vi "电机控制上位机 - 副本.vi"() -> ()   [LabVIEW 2018]
uses:
  <vilib>/Instr/_visa.llb/VISA Set IO Buffer Mask.ctl
  <vilib>/Instr/_visa.llb/VISA Configure Serial Port (Instr).vi
panel:
  in  "VISA resource name":refnum<visa-resource-name> caption="串口号"
  in  "目标速度Motor2":i16(slide) scale=-1000.0..1000.0
  in  "目标速度Motor1":i16(slide) step=100 scale=-1000.0..1000.0 scale format="%10d"
  out "数值 5":i32
  out "数值 4":u8
  out "无符号字节数组":u8[](array[numeric])
  out "数值 3":dbl
  out "布尔":bool
  out "目标速度2":i32
  out "值":enum32{"力矩模式", "速度模式", "位置模式"}(ring)
  in  "数值 2":i8
  in  "位置取反":bool
  out "目标速度 1":i32
  in  "弧度脉冲":bool
  out "数值":u8
  in  "运动控制":bool
  in  "串口设置":bool
  in  "示波器":bool
  in  "电机2":bool
  in  "电机1":bool
  in  "参数监控":bool
  in  "选项卡控件":T1(tab)
  in  "保存数据":bool
  in  "清空显示":bool
  out "字符串":string
  in  "参数下发":bool
  out "数      据      显      示":string
  in  "Flash保存":bool
  in  "串口号":refnum<visa-resource-name>="COM4"
  in  "波特率":u32(ring)=115200 items=["9600"=9600, "19200"=19200, "115200"=115200, "128000"=128000, "256000"=256000, "460800"=460800]
  in  "数据位":u16(ring)=8 items=["5"=5, "6"=6, "7"=7, "8"=8]
  in  "校验位":u16(ring) items=["None", "Odd", "Even", "Mark", "Space", ""]
  in  "停止位":u16(ring)=10 items=["1.0"=10, "1.5"=15, "2.0"=20]
  in  "打开/关闭串口":bool
  in  "参数上传":bool
  out "电机2状态":u32(ring) items=["无错误"=0, "FOC执行错误"=1, "过压"=2, "欠压"=4, "过温"=8, "霍尔错误"=16, "速度反馈错误"=32, "短路保护"=64, "软件错误"=128, "1_3倍过载"=256, "1_5倍过载"=512, "电机过流"=1024, "刹车电阻开启"=2048, "电机堵转"=4096, "电机失速"=8192, "位置跟随错误"=16384, "霍尔学习错误"=32768, "CAN通信错误"=65536, "电机缺相"=131072]
  out "电机2温度":i32(slide) scale=0.0..150.0
  out "电机1温度":i32(slide) scale=0.0..150.0
  out "母线电压":i32(knob) scale=0.0..50.0
  out "电机2实际位置":i32(knob) scale=-2147483647.0..2147483647.0
  out "电机2实际电流":i32(knob) scale=-20000.0..20000.0
  out "电机2实际速度":i32(knob) scale=-5000.0..5000.0
  out "电机1实际位置":i32(knob) scale=-2147483647.0..2147483647.0
  out "电机1实际电流":i32(knob) scale=-20000.0..20000.0
  out "电机1实际速度":i32(knob) scale=-5000.0..5000.0
  out "电机1状态":u32(ring) items=["无错误"=0, "FOC执行错误"=1, "过压"=2, "欠压"=4, "过温"=8, "霍尔错误"=16, "速度反馈错误"=32, "短路保护"=64, "软件错误 "=128, "1_3倍过载"=256, "1_5倍过载"=512, "电机过流"=1024, "刹车电阻开启"=2048, "电机堵转"=4096, "电机失速"=8192, "位置跟随错误"=16384, "霍尔学习错误"=32768, "CAN通信错误"=65536, "电机缺相"=131072]
  in  "写入3":bool
  in  "读取 3":bool
  in  "ID 3":u8
  in  "数值3":i32 caption="数值"
  in  "DIV1":u32
  in  "锁相环1":bool
  in  "Ppll":u32
  in  "Ipll":u32
  in  "发送保护参数":bool
  in  "堵转时间":i32
  in  "堵转电流":i32
  in  "堵转速度":i32
  in  "最大速度":i32
  in  "最大相电流":i32
  in  "峰值电流持续时间":i32
  in  "电机峰值电流":i32
  in  "发送电机参数":bool
  in  "编码器分辨率":u32
  in  "额定转速":i32
  in  "额定转矩":i32
  in  "额定电流":i32
  in  "电机惯量":i32
  in  "力矩常数":i32
  in  "Pairs":i32
  in  "Pc1":u32
  in  "Ic 1":u32
  in  "Pv1":u32
  in  "Iv 1":u32
  in  "Pp 1":u32
  in  "Ip 1":u32
  in  "发送 PID 1":bool
  in  "Dp1":u32
  in  "写入2":bool
  in  "读取 2":bool
  in  "ID 2":u8
  in  "数值2":i32 caption="数值"
  in  "DIV2":u32
  in  "锁相环2":bool
  in  "Ppll 2":u32 caption="Ppll"
  in  "Ipll 2":u32
  in  "Dp2":u32
  in  "发送 PID 2":bool
  in  "Ip 2":u32
  in  "Pp2":u32
  in  "Iv 2":u32
  in  "Pv 2":u32
  in  "Ic2":u32
  in  "Pc 2":u32
  in  "Pairs 2":i32
  in  "力矩常数 2":i32
  in  "电机惯量 2":i32
  in  "额定电流 2":i32
  in  "额定转矩 2":i32
  in  "额定转速 2":i32
  in  "编码器分辨率 2":i32
  in  "发送电机参数 2":bool
  in  "电机峰值电流 2":i32
  in  "峰值电流持续时间 2":i32
  in  "最大相电流 2":i32
  in  "最大速度 2":i32
  in  "堵转速度 2":i32
  in  "堵转电流 2":i32
  in  "堵转时间 2":i32
  in  "发送保护参数 2":bool
  in  "同步模式开关":bool
  in  "写入":bool
  in  "读取":bool
  in  "ID":u8
  in  "数值1":i32 caption="数值"
  in  "确认换向参数":bool
  in  "换向电流":i32
  in  "确认电机":bool
  in  "确定运行模式":bool
  in  "执行换向":bool
  in  "电机失能":bool
  in  "运行模式":enum32{"力矩模式", "速度模式", "位置模式"}(tab)
  in  "目标力矩Motor 2":i32
  in  "下发力矩参数":bool
  in  "目标力矩Motor 1":i32
  in  "目标时间Motor2":i32
  in  "目标速度Motor2":i32
  in  "目标时间Motor1":i32
  in  "目标速度Motor1":i32
  in  "下发速度参数":bool
  in  "目标位置Motor2":i32
  in  "目标加速度Motor2":i32
  in  "目标减速度Motor2":i32
  in  "目标速度Motor2":i32
  in  "下发位置参数":bool
  in  "目标位置Motor1":i32
  in  "目标加速度Motor1":i32
  in  "目标减速度Motor1":i32
  in  "目标速度Motor1":i32
  in  "换向模式":string(combo)="1"
  in  "Motor1":bool
  in  "Motor2":bool
  in  "电机使能":bool
  in  "急停":bool
  in  "运行模式1":string(combo)="2"
  out "数值1 2":i32 caption="数值" format="%x"
  in  "报警清除":bool
  in  "参数确定":bool
  in  "确认ID":bool
  in  "参数4":u8(ring) items=["电机1参考电流", "电机1实际电流", "电机1参考速度", "电机1实际速度", "电机1参考位置", "电机1实际位置", "电机2参考电流", "电机2实际电流", "电机2参考速度", "电机2实际速度", "电机2参考位置", "电机2实际位置", ""]
  in  "参数3":u8(ring) items=["电机1参考电流", "电机1实际电流", "电机1参考速度", "电机1实际速度", "电机1参考位置", "电机1实际位置", "电机2参考电流", "电机2实际电流", "电机2参考速度", "电机2实际速度", "电机2参考位置", "电机2实际位置", ""]
  in  "参数2":T2(ring)
  in  "参数1":u8(ring) items=["电机1参考电流", "电机1实际电流", "电机1参考速度", "电机1实际速度", "电机1参考位置", "电机1实际位置", "电机2参考电流", "电机2实际电流", "电机2参考速度", "电机2实际速度", "电机2参考位置", "电机2实际位置", ""]
  in  "ID 4":u8
  in  "ID 3":u8
  in  "ID 2":u8
  in  "ID 1":u8
  out "波形图表":cluster{i32, i32, i32, i32}(graph)
  in  "停止":bool
  # "电机极对数"
  # "pairs"
  # "峰值电流"
  # "mA"
  # "mNm/A"
  # "ms"
  # "力矩常数"
  # "峰值时间"
  # "电机惯量"
  # "Kgm2"
  # "最大相电流"
  # "mA"
  # "rpm"
  # "额定电流"
  # "mA"
  # "最大速度"
  # "mNm"
  # "rpm"
  # "额定转矩"
  # "堵转速度"
  # "额定转速"
  # "rpm"
  # "堵转电流"
  # "mA"
  # "编码器分辨率"
  # "counts/r"
  # "堵转时间"
  # "ms"
  # "电流环"
  # "Pc"
  # "位置环"
  # "Ppll"
  # "Pp"
  # "Ic"
  # "Ip"
  # "Ipll"
  # "速度环"
  # "DIV"
  # "Dp"
  # "Pv"
  # "Iv"
  # "独立参数读取"
  # "pairs"
  # "mA"
  # "电机极对数"
  # "峰值电流"
  # "mNm/A"
  # "力矩常数"
  # "ms"
  # "峰值时间"
  # "Kgm2"
  # "电机惯量"
  # "mA"
  # "最大相电流"
  # "mA"
  # "rpm"
  # "额定电流"
  # "最大速度"
  # "mNm"
  # "额定转矩"
  # "rpm"
  # "堵转速度"
  # "rpm"
  # "额定转速"
  # "mA"
  # "堵转电流"
  # "counts/r"
  # "编码器分辨率"
  # "ms"
  # "堵转时间"
  # "电流环"
  # "位置环"
  # "Pc"
  # "Pp"
  # "Ppll"
  # "Ic"
  # "Ip"
  # "速度环"
  # "Ipll"
  # "Pv"
  # "Dp"
  # "DIV"
  # "Iv"
  # "独立参数读取"
  # "电机选择"
  # "独立参数读取"
  # "mA"
  # "mNm"
  # "mNm"
  # "rpm"
  # "ms"
  # "rpm"
  # "ms"
  # "counts"
  # "counts"
  # "rpm"
  # "rpm"
  # "rpm/s"
  # "rpm/s"
  # "rpm/s"
  # "rpm/s"
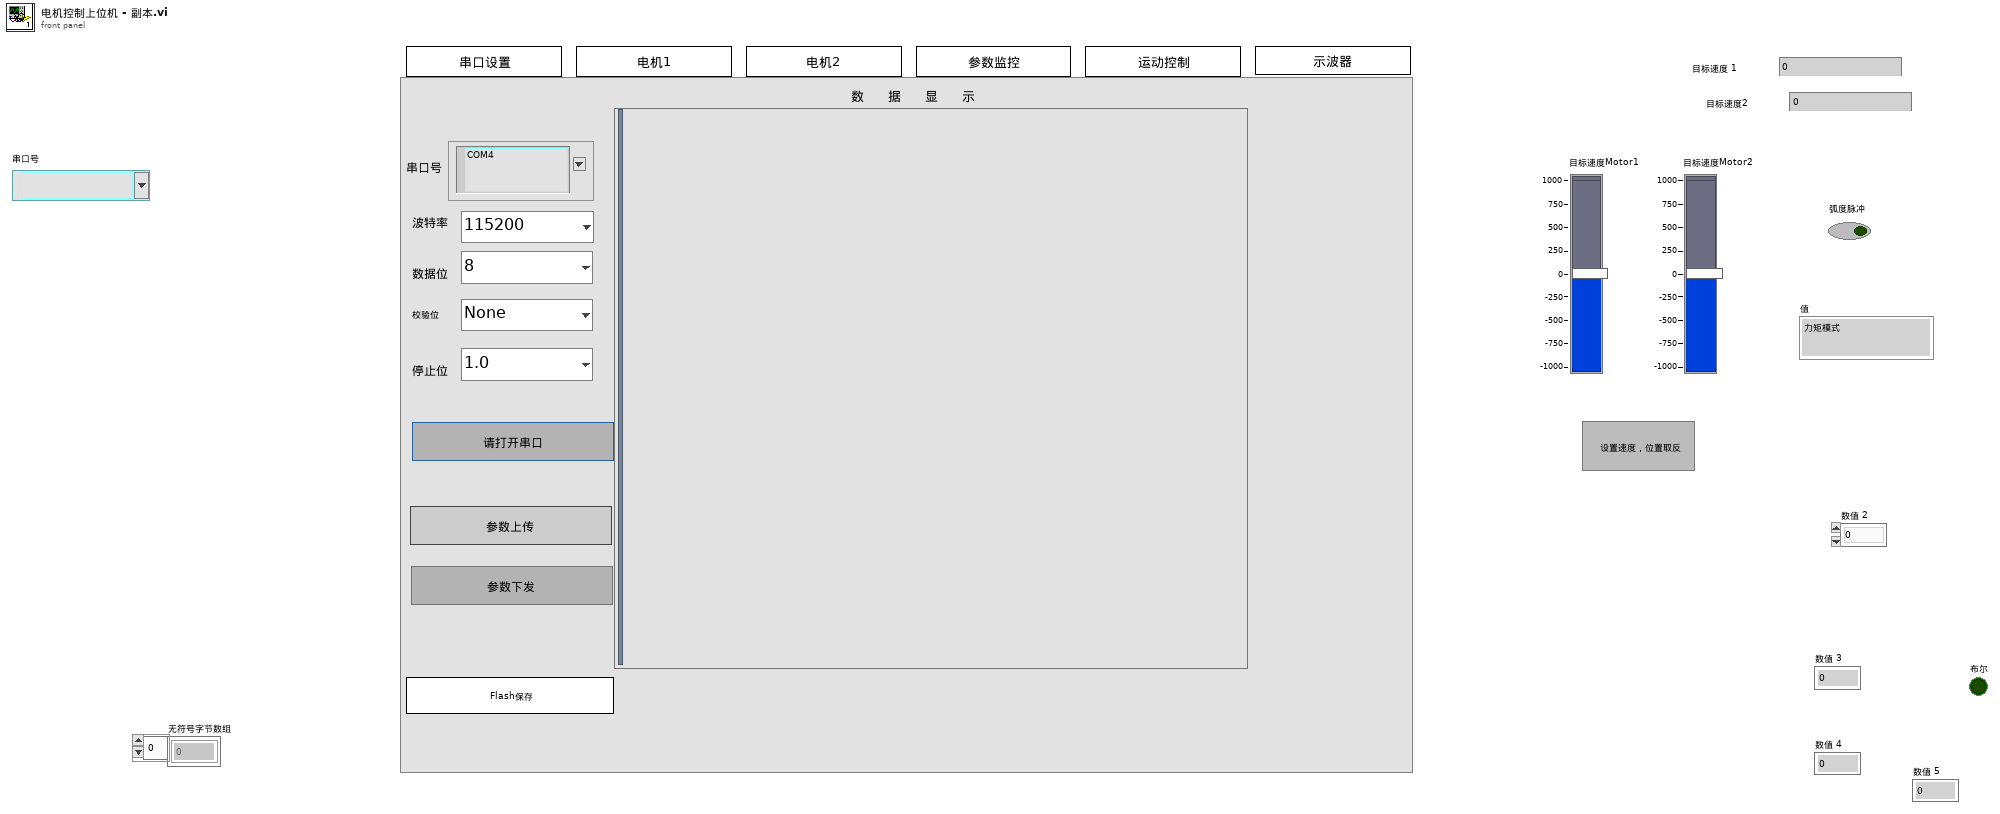
[diagram p1: front panel]
types:
  T1 = enum32{"串口设置", "参数监控", "电机1", "电机2", "运动控制", "示波器"}
  T2 = enum8{"电机1参考电流", "电机1实际电流", "电机1参考速度", "电机1实际速度", "电机1参考位置", "电机1实际位置", "电机2参考电流", "电机2实际电流", "电机2参考速度", "电机2实际速度", "电机2参考位置", "电机2实际位置", ""}
  T3 = enum16{"open", "replace", "create", "open or create", "replace or create", "replace or create with confirmation"}
  T4 = typedef "VISA Set IO Buffer Mask.ctl" = u16
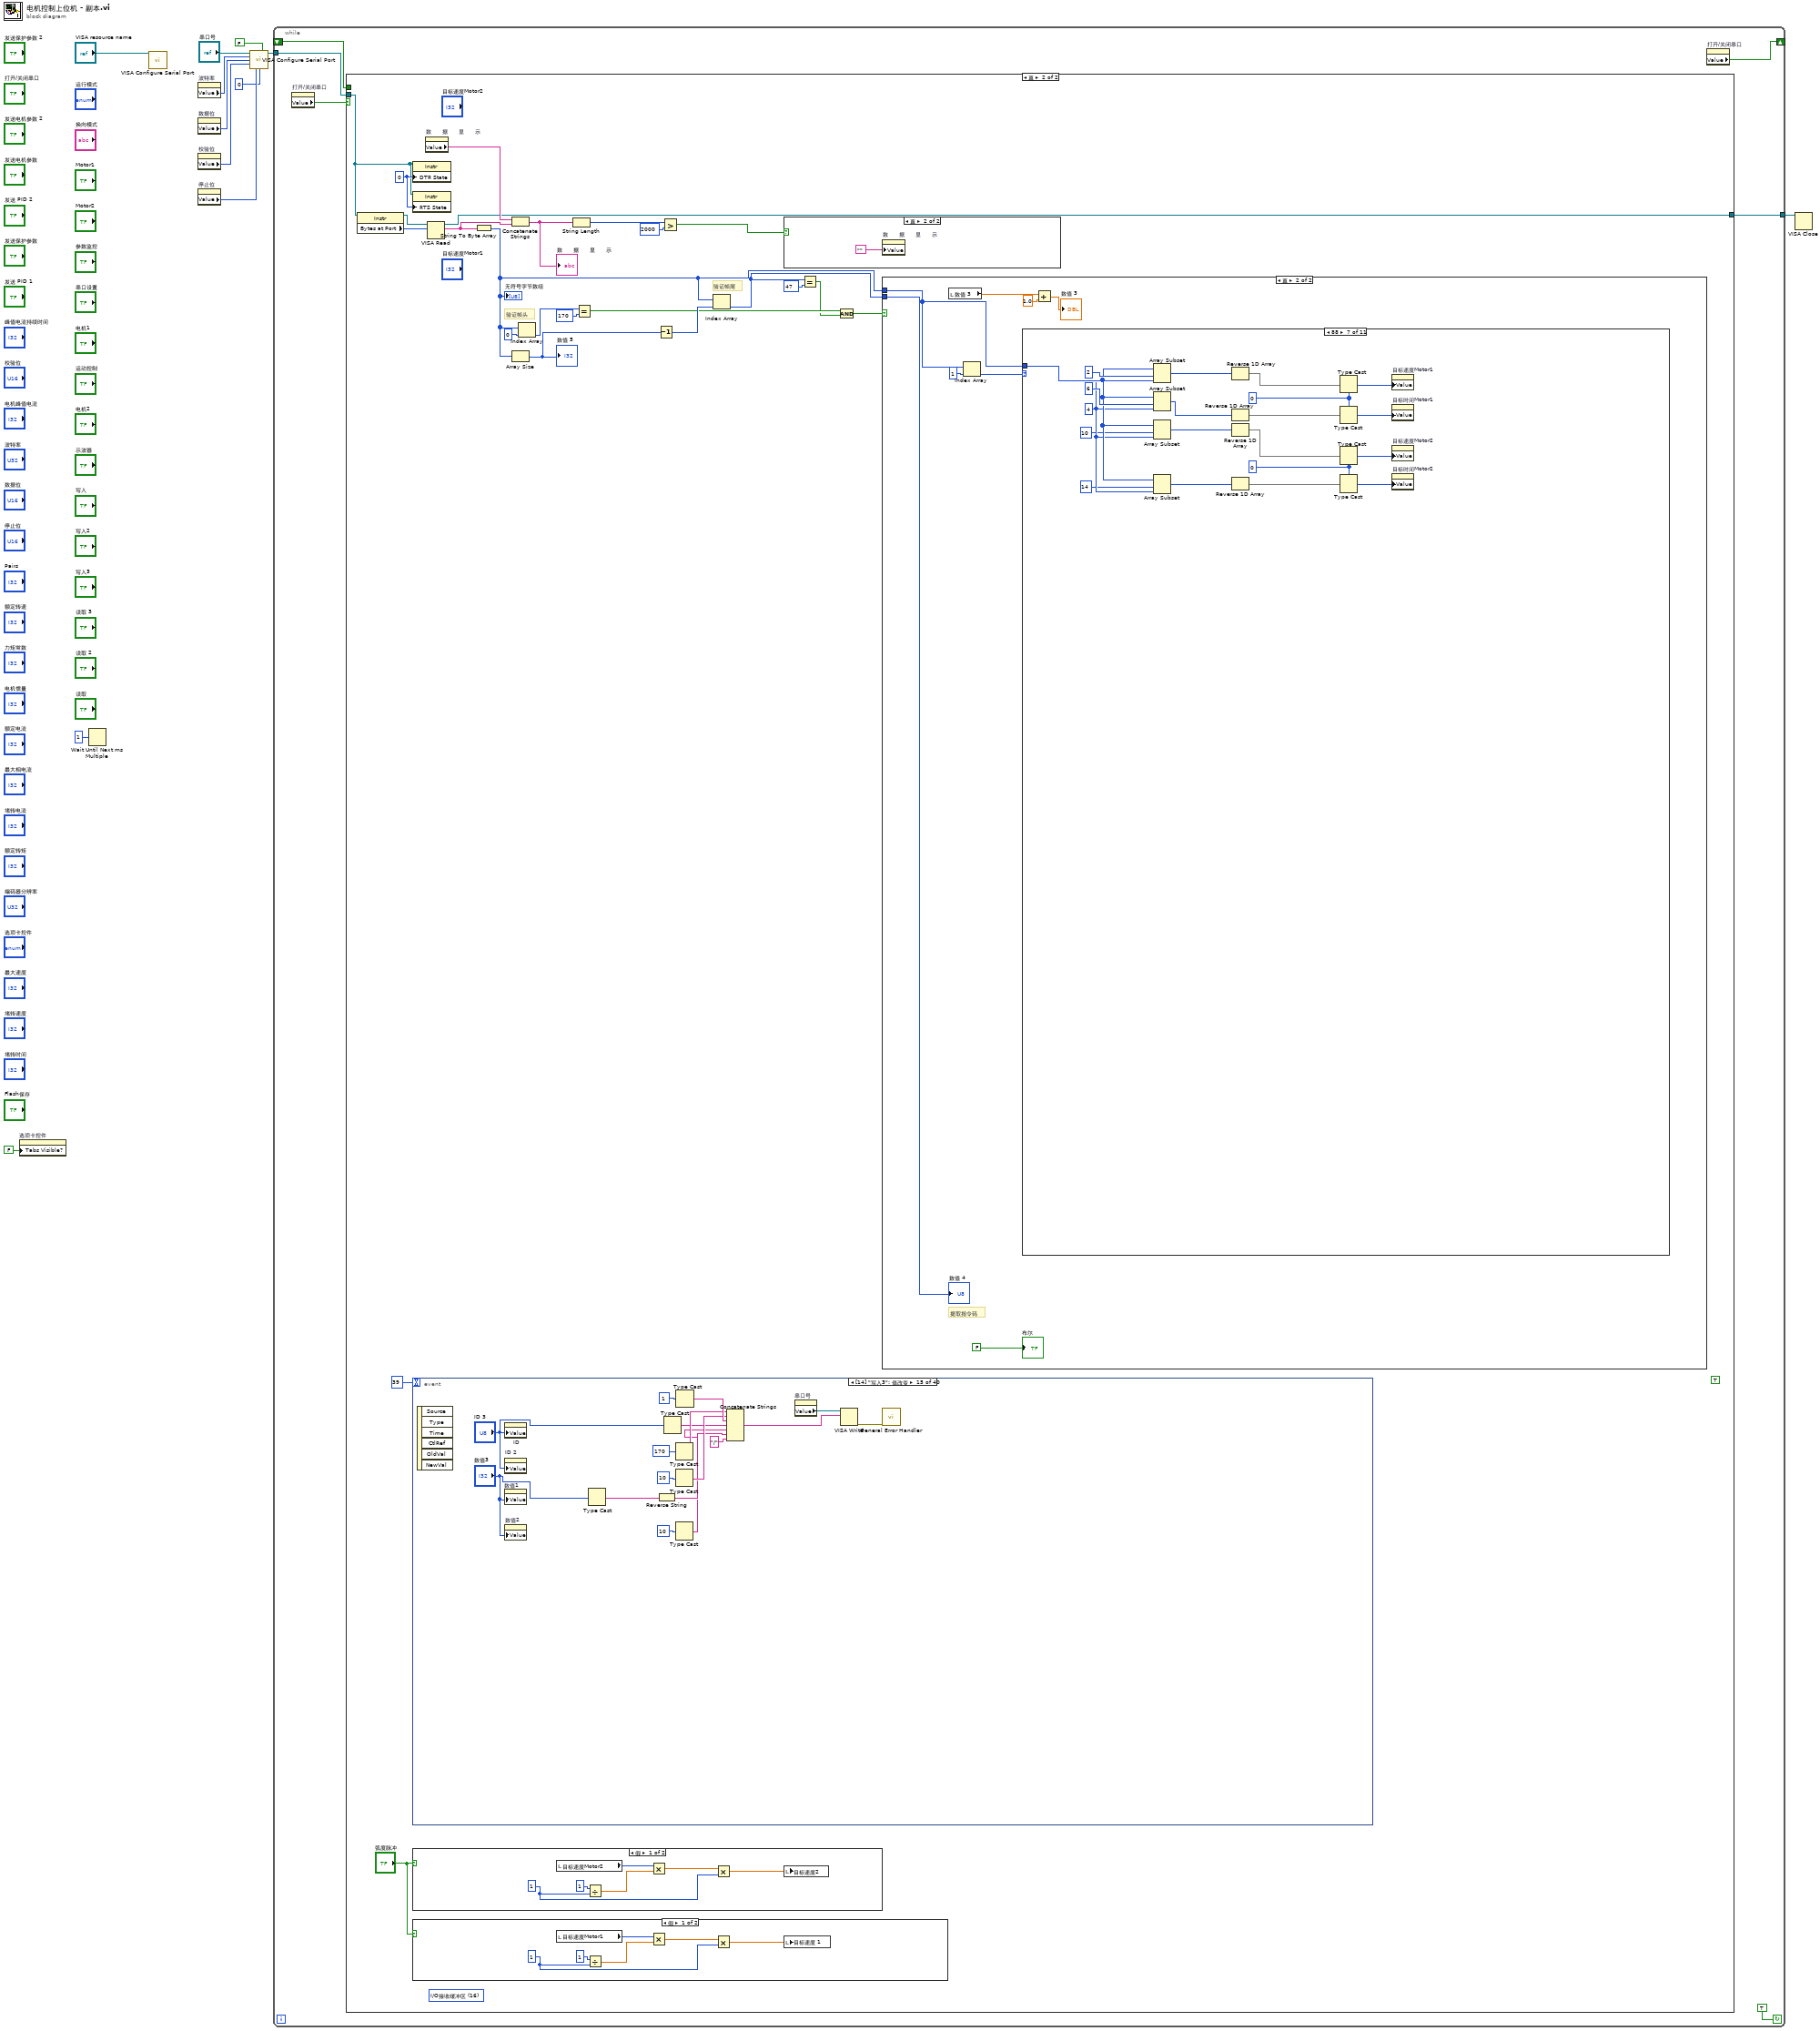
[diagram p0: block diagram]
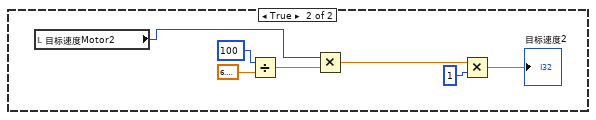
[diagram p3: hidden frame]
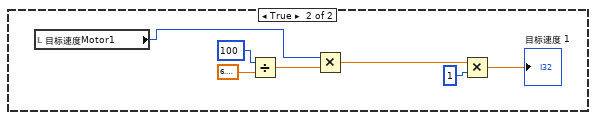
[diagram p5: hidden frame]
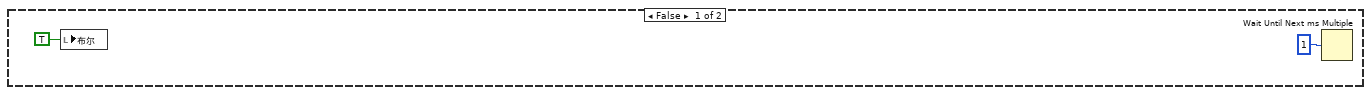
[diagram p6: hidden frame]
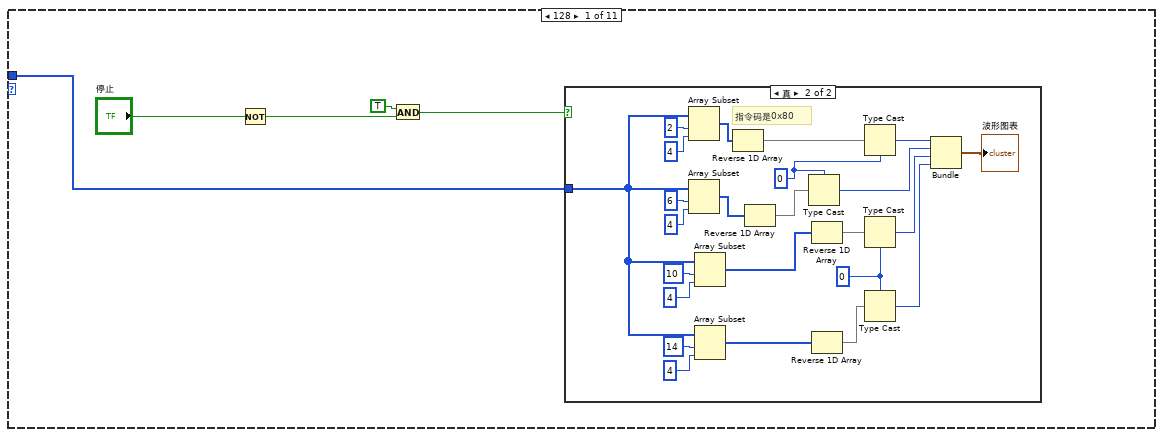
[diagram p7: hidden frame]
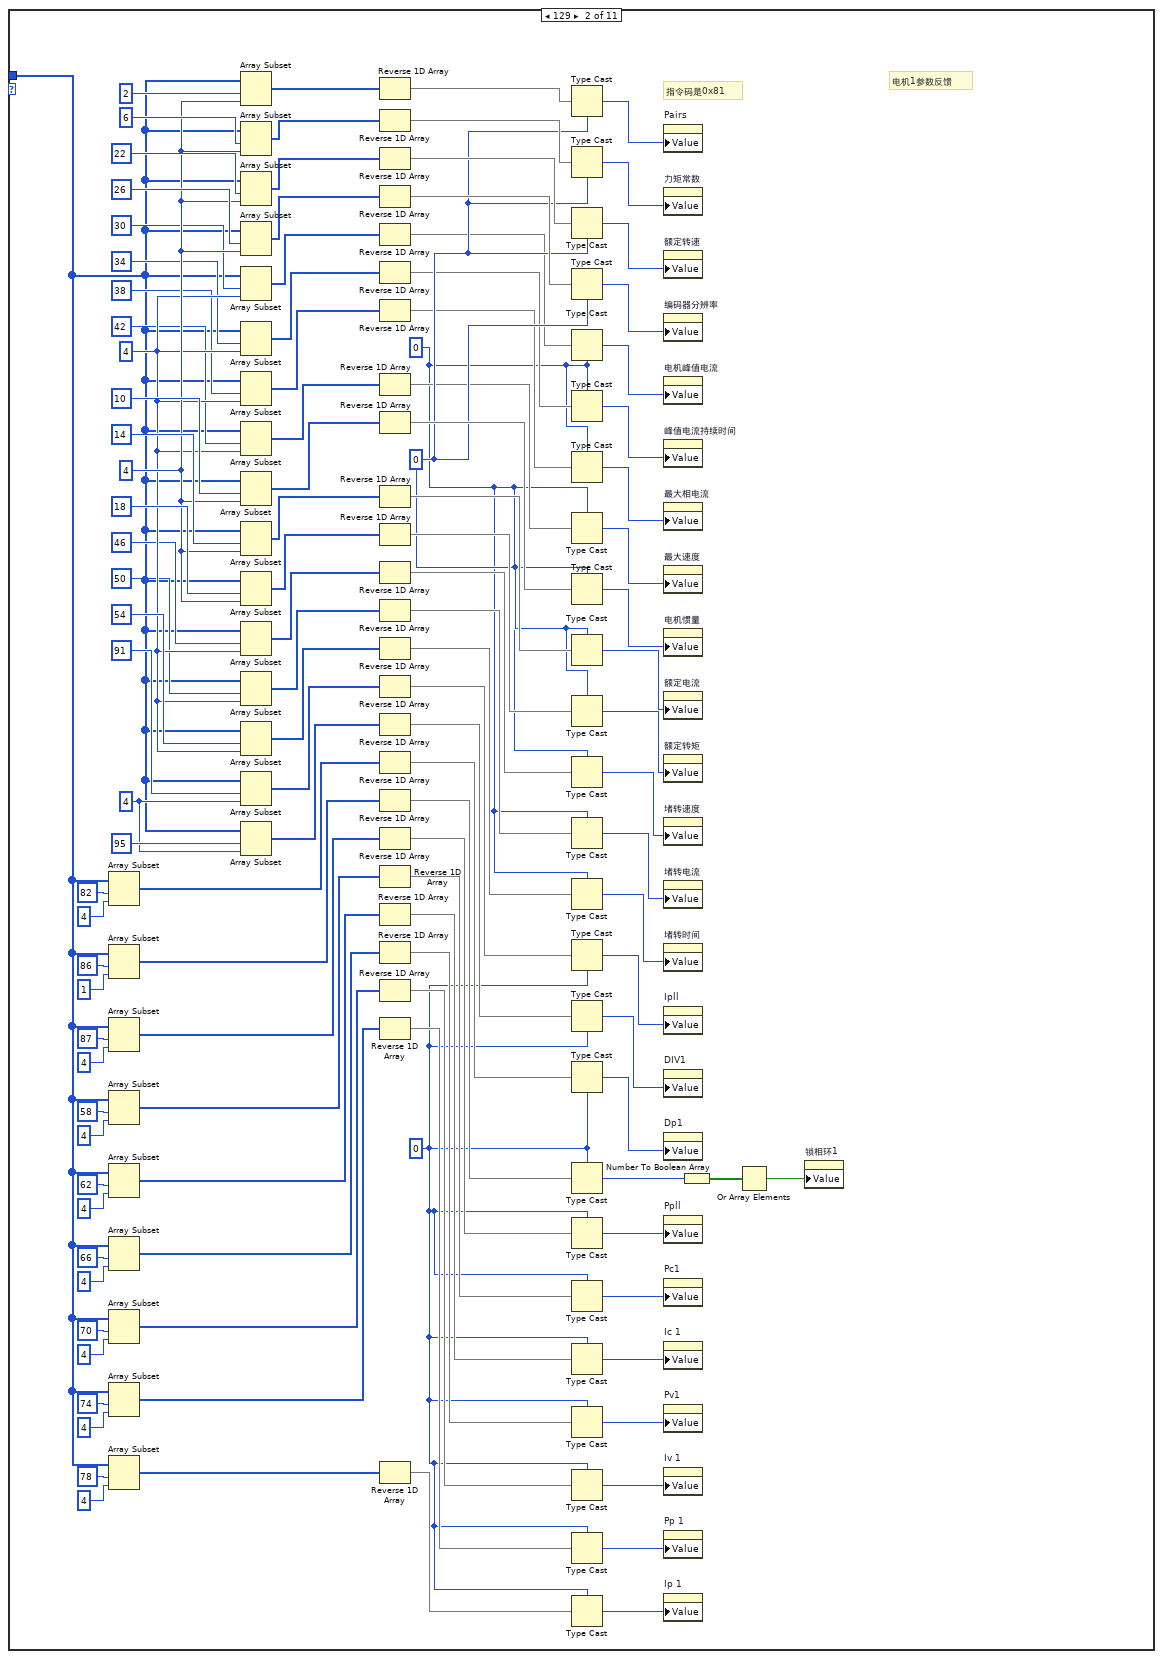
[diagram p9: hidden frame]
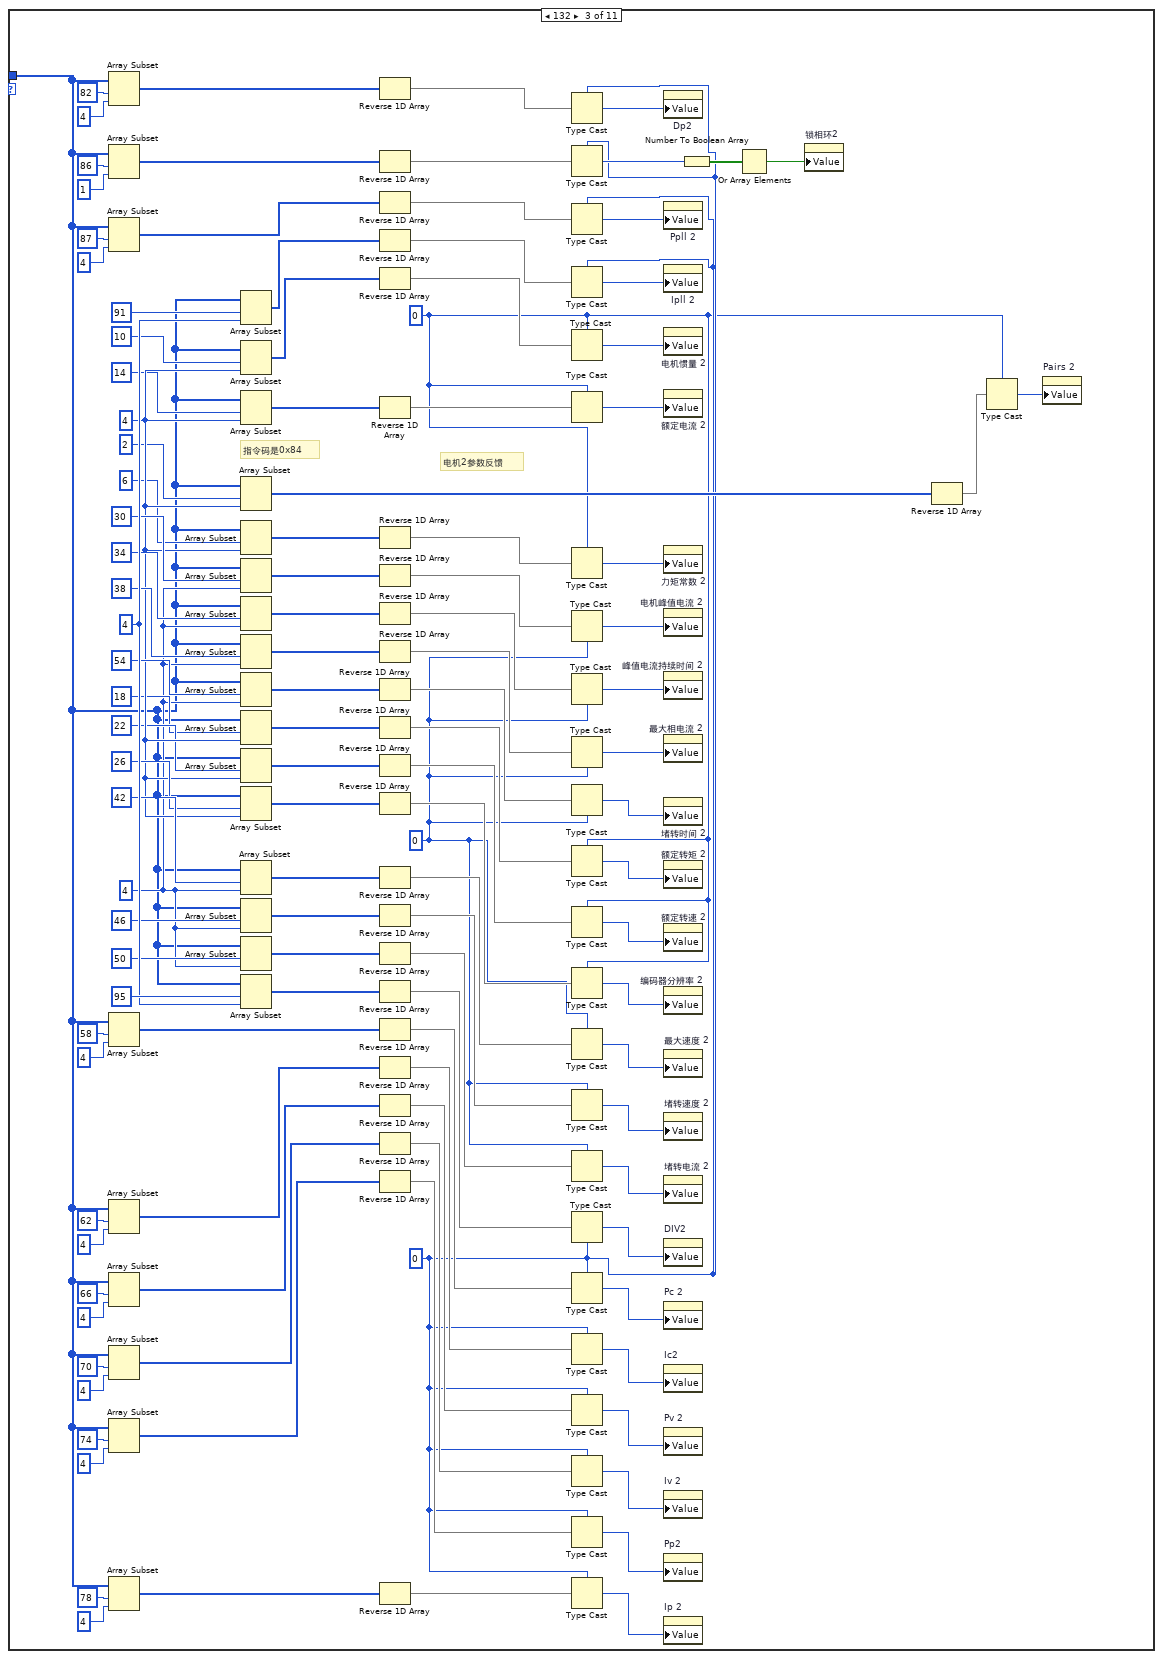
[diagram p10: hidden frame]
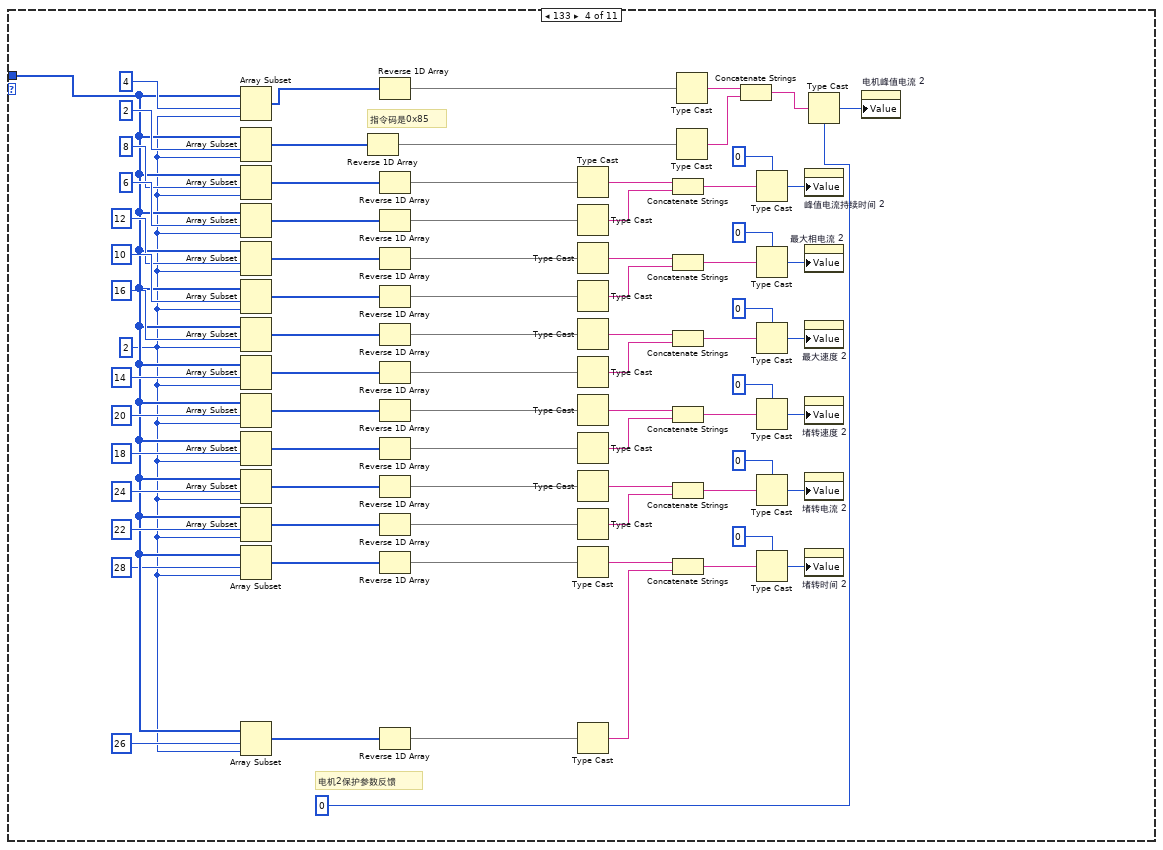
[diagram p11: hidden frame]
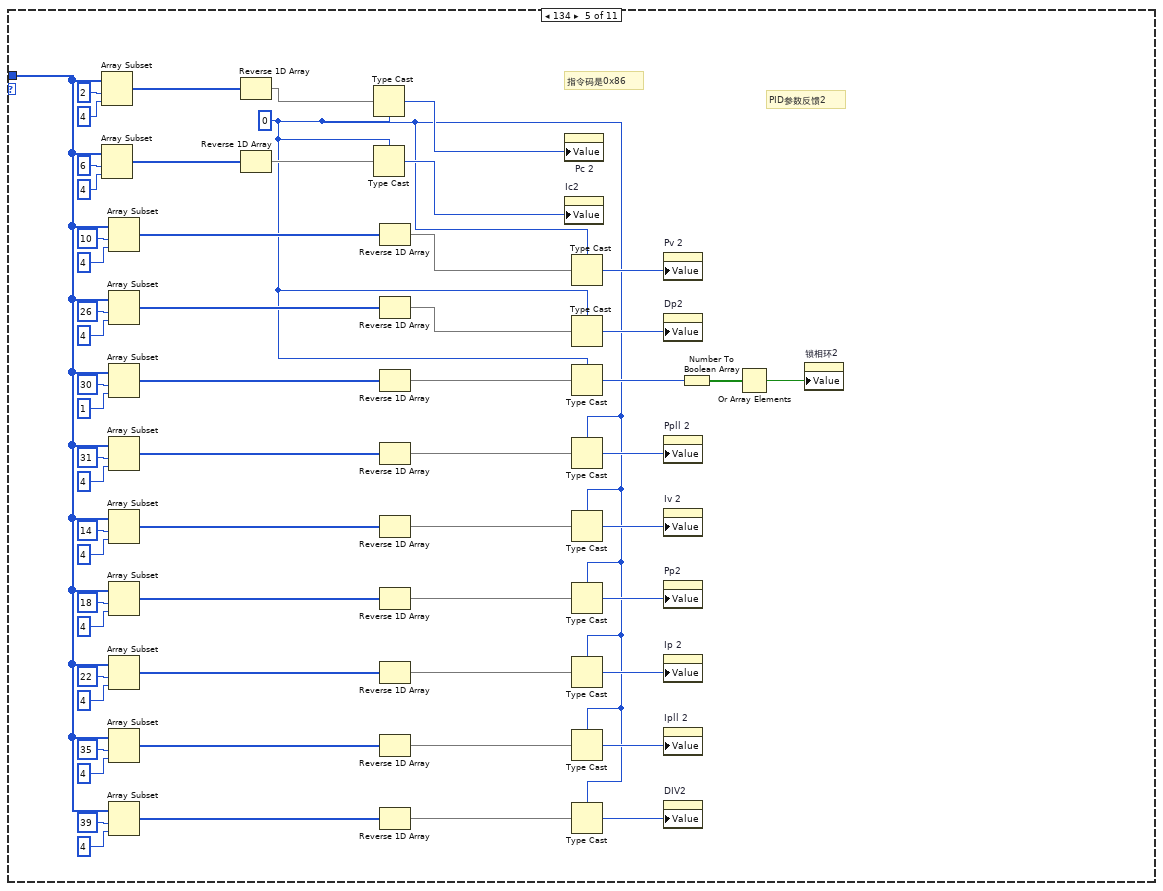
[diagram p12: hidden frame]
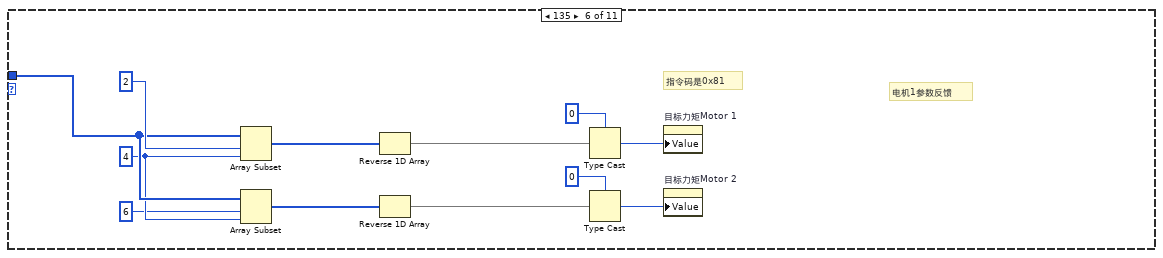
[diagram p13: hidden frame]
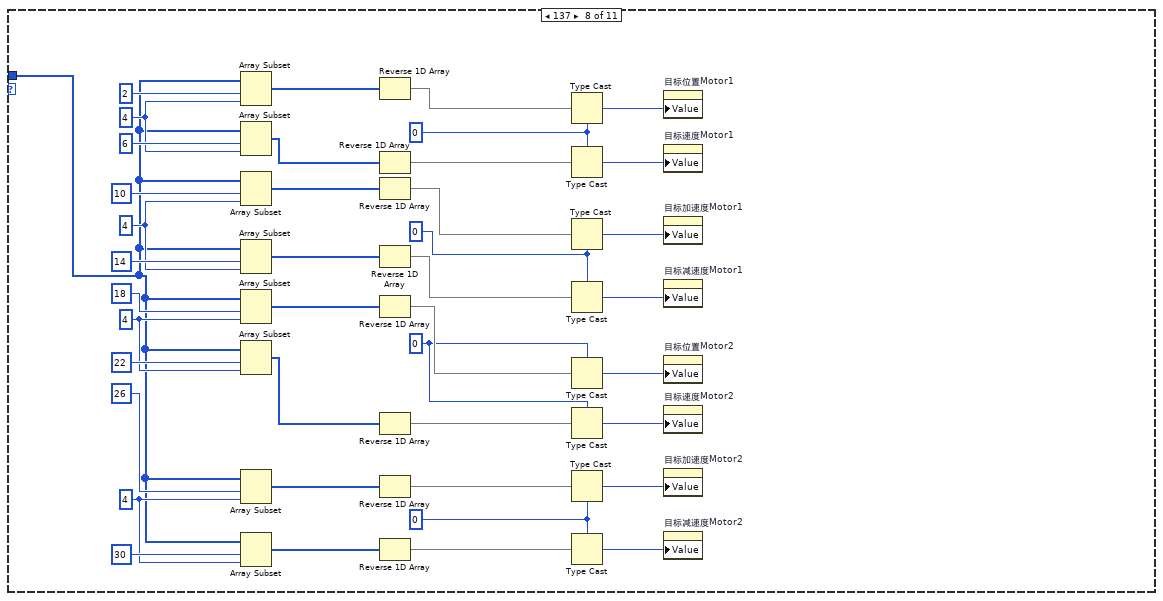
[diagram p14: hidden frame]
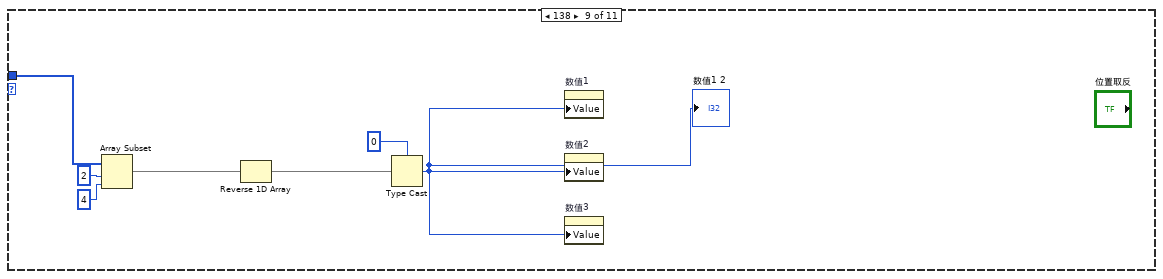
[diagram p15: hidden frame]
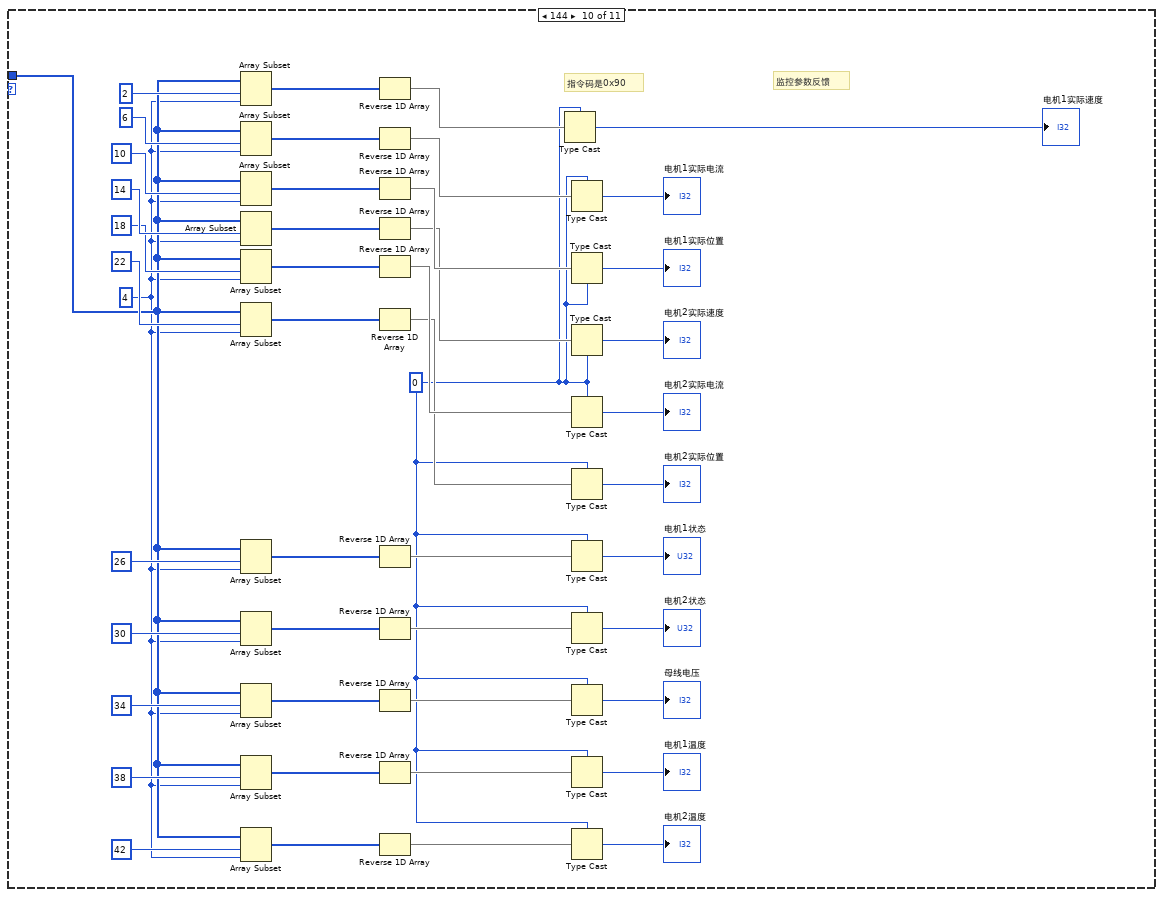
[diagram p16: hidden frame]
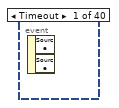
[diagram p18: hidden frame]
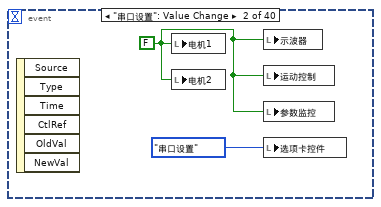
[diagram p19: hidden frame]
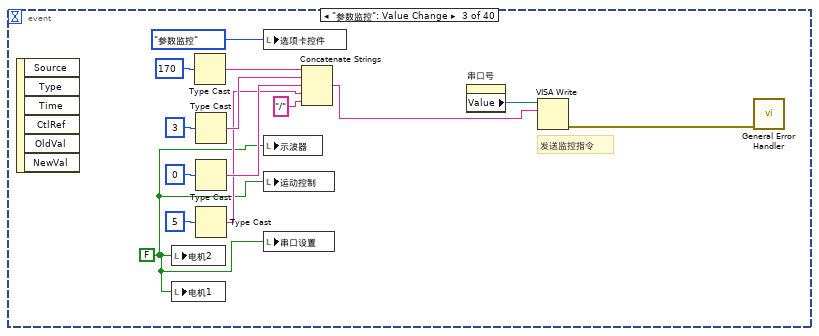
[diagram p20: hidden frame]
diagram:
  n1 = property on="选项卡控件" class="TabCtl (严格)"("Tabs Visible?"=FALSE) -> ()  [unwired: 2 in, 2 out]
  n2 = Wait Until Next ms Multiple(millisecond multiple=1) -> ()  [unwired: 1 out]
  n3 = call-poly "VISA Configure Serial Port"("VISA resource name"="VISA resource name") -> ()  [unwired: 13 in, 2 out]
  n4 = property on="波特率" class="Ring (严格)"() -> ("Value"=w2:u32)  [unwired: 2 in, 2 out]
  n5 = property on="数据位" class="Ring (严格)"() -> ("Value"=w8:u16)  [unwired: 2 in, 2 out]
  n6 = property on="校验位" class="Ring (严格)"() -> ("Value"=w9:u16)  [unwired: 2 in, 2 out]
  n7 = property on="停止位" class="Ring (严格)"() -> ("Value"=w10:u16)  [unwired: 2 in, 2 out]
  n8 = call-poly "VISA Configure Serial Port"("VISA resource name"="串口号", "Enable Termination\nChar (T)"=FALSE ("Enable Termination\nChar (T)"), "baud rate (9600)"=w2, "data bits (8)"=w8, "parity (0:none)"=w9, "stop bits (10: 1 bit)"=w10, "flow control (0:none)"=0) -> ("VISA resource name out"=w4:refnum<visa-resource-name>)  [unwired: 7 in, 1 out]
  n9 = while {
    shift-right: [w16] -> _
    shift-left: _ -> [w15]
    tunnel: w4 -> [w14]
    tunnel: [w13] -> w5
    stop <- TRUE continue-if-true
    n10 = property on="打开/关闭串口" class="Bool (严格)"() -> ("Value"=w18:bool)  [unwired: 2 in, 2 out]
    n11 = case shown="真" w18 {
      tunnel: w15 -> [_ _]
      tunnel: w14 -> [_ w20]
      tunnel: [_ w19] -> w13
      frame False {
      }
      frame True {
        (unwired) T4 16 items=["I/O接收缓冲区"=16, "I/O传输缓冲区"=32, "I/O接收和传输缓冲区"=48] ("Mask")
        (unwired) TRUE ("布尔")
        w42 = 0
        # "验证帧尾"
        # "验证帧头"
        n12 = property class="Instr"(reference=w20) -> (reference out=w34:refnum<visa-resource-name>, "Bytes at Port"=w41:u32)  [unwired: 1 in, 1 out]
        n13 = property class="Instr"(reference=w20, "DTR State"=w42) -> ()  [unwired: 1 in, 2 out]
        n14 = property class="Instr"(reference=w20, "RTS State"=w42) -> ()  [unwired: 1 in, 2 out]
        n15 = event shown="[14] \"写入3\": 值改变" {
          selector: _ -> [_ _ _ _ _ _ _ _ _ _ _ _ _ _ _ _ _ _ _ _ _ _ _ _ _ _ _ _ _ _ _ _ _ _ _ _ _ _ _ _]
          dyn-events: _ -> [_ _ _ _ _ _ _ _ _ _ _ _ _ _ _ _ _ _ _ _ _ _ _ _ _ _ _ _ _ _ _ _ _ _ _ _ _ _ _ _]
          timeout: 39 -> [_ _ _ _ _ _ _ _ _ _ _ _ _ _ _ _ _ _ _ _ _ _ _ _ _ _ _ _ _ _ _ _ _ _ _ _ _ _ _ _]
          event Timeout {
            n16 = event-data() -> ()  [unwired: 1 in, 2 out]
          }
          event "串口设置": Value Change {
            w610 = FALSE
            n17 = event-data() -> ()  [unwired: 1 in, 6 out]
            n18 = local write "电机1"(w610) -> ()
            n19 = local write "电机2"(w610) -> ()
            n20 = local write "示波器"(w610) -> ()
            n21 = local write "运动控制"(w610) -> ()
            n22 = local write "参数监控"(w610) -> ()
            n23 = local write "选项卡控件"(T1."串口设置" ("选项卡控件")) -> ()
          }
          event "参数监控": Value Change {
            w612 = FALSE
            # "发送监控指令"
            n24 = event-data() -> ()  [unwired: 1 in, 6 out]
            n25 = local write "电机2"(w612) -> ()
            n26 = local write "电机1"(w612) -> ()
            n27 = Type Cast(x=u8 170) -> (*(type *) &x=w621:string)  [unwired: 1 in]
            n28 = Type Cast(x=u8 3) -> (*(type *) &x=w622:string)  [unwired: 1 in]
            n29 = Type Cast(x=u8 0) -> (*(type *) &x=w618:string)  [unwired: 1 in]
            n30 = Type Cast(x=u8 5) -> (*(type *) &x=w613:string)  [unwired: 1 in]
            n31 = local write "选项卡控件"(T1."参数监控" ("选项卡控件")) -> ()
            n32 = local write "示波器"(w612) -> ()
            n33 = local write "运动控制"(w612) -> ()
            n34 = local write "串口设置"(w612) -> ()
            n35 = Concatenate Strings(w621, w622, w618, w613, "/") -> (w623:string)
            n36 = property on="串口号" class="VISAName"() -> ("Value"=w617:refnum<visa-resource-name>)  [unwired: 2 in, 2 out]
            n37 = VISA Write(VISA resource name=w617, write buffer=w623) -> (error out=w624:errorcluster)  [unwired: 1 in, 2 out]
            n38 = call <vilib>:"General Error Handler.vi"("error in (no error)"=w624) -> ()  [unwired: 10 in, 5 out]
          }
          event "报警清除": Value Change {
            n39 = event-data() -> ("OldVal"=w628:bool, "NewVal"=w627:bool)  [unwired: 1 in, 4 out]
            n40 = Not(x=w628) -> (.not. x?=w629:bool)
            n41 = And(x=w629, y=w627) -> ()  [unwired: 1 out]
            n42 = case shown="真" "报警清除" {
              frame False {
              }
              frame True {
                n43 = Type Cast(x=u8 170) -> (*(type *) &x=w637:string)  [unwired: 1 in]
                n44 = Type Cast(x=u8 9) -> (*(type *) &x=w638:string)  [unwired: 1 in]
                n45 = Type Cast(x=u8 0) -> (*(type *) &x=w634:string)  [unwired: 1 in]
                n46 = Type Cast(x=u8 5) -> (*(type *) &x=w630:string)  [unwired: 1 in]
                n47 = Concatenate Strings(w637, w638, w634, w630, "/") -> (w639:string)
                n48 = property on="串口号" class="VISAName"() -> ("Value"=w633:refnum<visa-resource-name>)  [unwired: 2 in, 2 out]
                n49 = VISA Write(VISA resource name=w633, write buffer=w639) -> (error out=w640:errorcluster)  [unwired: 1 in, 2 out]
                n50 = call <vilib>:"General Error Handler.vi"("error in (no error)"=w640) -> ()  [unwired: 10 in, 5 out]
              }
            }
          }
          event "电机1": Value Change {
            n51 = event-data() -> ("OldVal"=w648:bool, "NewVal"=w647:bool)  [unwired: 1 in, 4 out]
            n52 = Not(x=w648) -> (.not. x?=w650:bool)
            n53 = local write "电机2"(FALSE) -> ()
            n54 = local write "示波器"(FALSE) -> ()
            n55 = local write "运动控制"(FALSE) -> ()
            n56 = local write "参数监控"(FALSE) -> ()
            n57 = local write "串口设置"(FALSE) -> ()
            n58 = local write "选项卡控件"(T1."电机1" ("选项卡控件")) -> ()
            n59 = And(x=w650, y=w647) -> (x .and. y?=w649:bool)
            n60 = case shown="真" w649 {
              frame False {
              }
              frame True {
                n61 = Type Cast(x=u8 170) -> (*(type *) &x=w661:string)  [unwired: 1 in]
                n62 = Type Cast(x=u8 1) -> (*(type *) &x=w660:string)  [unwired: 1 in]
                n63 = Type Cast(x=u8 0) -> (*(type *) &x=w662:string)  [unwired: 1 in]
                n64 = Type Cast(x=u8 5) -> (*(type *) &x=w653:string)  [unwired: 1 in]
                n65 = Concatenate Strings(w661, w660, w662, w653, "/") -> (w659:string)
                n66 = property on="串口号" class="VISAName"() -> ("Value"=w663:refnum<visa-resource-name>)  [unwired: 2 in, 2 out]
                n67 = VISA Write(VISA resource name=w663, write buffer=w659) -> (error out=w658:errorcluster)  [unwired: 1 in, 2 out]
                n68 = call <vilib>:"General Error Handler.vi"("error in (no error)"=w658) -> ()  [unwired: 10 in, 5 out]
              }
            }
          }
          event "电机2": Value Change {
            w664 = FALSE
            n69 = event-data() -> ("OldVal"=w667:bool, "NewVal"=w668:bool)  [unwired: 1 in, 4 out]
            n70 = Not(x=w667) -> (.not. x?=w669:bool)
            n71 = local write "电机1"(w664) -> ()
            n72 = local write "选项卡控件"(T1."电机2" ("选项卡控件")) -> ()
            n73 = And(x=w669, y=w668) -> (x .and. y?=w666:bool)
            n74 = local write "参数监控"(w664) -> ()
            n75 = local write "示波器"(w664) -> ()
            n76 = local write "运动控制"(w664) -> ()
            n77 = local write "串口设置"(w664) -> ()
            n78 = case shown="真" w666 {
              frame False {
              }
              frame True {
                n79 = Type Cast(x=u8 170) -> (*(type *) &x=w677:string)  [unwired: 1 in]
                n80 = Type Cast(x=u8 2) -> (*(type *) &x=w678:string)  [unwired: 1 in]
                n81 = Type Cast(x=u8 0) -> (*(type *) &x=w675:string)  [unwired: 1 in]
                n82 = Type Cast(x=u8 5) -> (*(type *) &x=w671:string)  [unwired: 1 in]
                n83 = Concatenate Strings(w677, w678, w675, w671, "/") -> (w679:string)
                n84 = property on="串口号" class="VISAName"() -> ("Value"=w673:refnum<visa-resource-name>)  [unwired: 2 in, 2 out]
                n85 = VISA Write(VISA resource name=w673, write buffer=w679) -> (error out=w680:errorcluster)  [unwired: 1 in, 2 out]
                n86 = call <vilib>:"General Error Handler.vi"("error in (no error)"=w680) -> ()  [unwired: 10 in, 5 out]
              }
            }
          }
          event "运动控制": Value Change {
            w682 = FALSE
            n87 = event-data() -> ()  [unwired: 1 in, 6 out]
            n88 = local write "电机2"(w682) -> ()
            n89 = local write "电机1"(w682) -> ()
            n90 = local write "参数监控"(w682) -> ()
            n91 = local write "示波器"(w682) -> ()
            n92 = local write "串口设置"(w682) -> ()
            n93 = local write "选项卡控件"(T1."运动控制" ("选项卡控件")) -> ()
          }
          event "执行换向": Value Change {
            n94 = event-data() -> ()  [unwired: 1 in, 6 out]
            n95 = property on="换向模式" class="CmbBox"() -> ("Value"=w697:string)  [unwired: 2 in, 2 out]
            n96 = case shown="\"2\"" w697 {
              tunnel: [i8 1 i8 2] -> w696
              frame "1", Default {
              }
              frame "2" {
              }
            }
            n97 = property on="数值" class="DigNum (严格)"() -> ("Value"=w698:u8)  [unwired: 2 in, 2 out]
            n98 = Type Cast(x=w698) -> (*(type *) &x=w689:string)  [unwired: 1 in]
            n99 = Type Cast(x=w696) -> (*(type *) &x=w687:string)  [unwired: 1 in]
            n100 = Type Cast(x=u8 170) -> (*(type *) &x=w695:string)  [unwired: 1 in]
            n101 = Type Cast(x=u8 7) -> (*(type *) &x=w694:string)  [unwired: 1 in]
            n102 = Type Cast(x=u8 6) -> (*(type *) &x=w685:string)  [unwired: 1 in]
            n103 = Concatenate Strings(w695, w694, w689, w687, w685, "/") -> (w693:string)
            n104 = property on="串口号" class="VISAName"() -> ("Value"=w688:refnum<visa-resource-name>)  [unwired: 2 in, 2 out]
            n105 = VISA Write(VISA resource name=w688, write buffer=w693) -> (error out=w692:errorcluster)  [unwired: 1 in, 2 out]
            n106 = call <vilib>:"General Error Handler.vi"("error in (no error)"=w692) -> ()  [unwired: 10 in, 5 out]
          }
          event "电机使能": Value Change {
            n107 = event-data() -> ()  [unwired: 1 in, 6 out]
            n108 = property on="数值" class="DigNum (严格)"() -> ("Value"=w701:u8)  [unwired: 2 in, 2 out]
            n109 = case shown="真" "电机使能" {
              tunnel: w701 -> [_ w706]
              frame False {
              }
              frame True {
                n110 = Type Cast(x=w706) -> (*(type *) &x=w708:string)  [unwired: 1 in]
                n111 = Type Cast(x=u8 170) -> (*(type *) &x=w714:string)  [unwired: 1 in]
                n112 = Type Cast(x=u8 4) -> (*(type *) &x=w713:string)  [unwired: 1 in]
                n113 = Type Cast(x=u8 5) -> (*(type *) &x=w703:string)  [unwired: 1 in]
                n114 = Concatenate Strings(w714, w713, w708, w703, "/") -> (w712:string)
                n115 = property on="串口号" class="VISAName"() -> ("Value"=w707:refnum<visa-resource-name>)  [unwired: 2 in, 2 out]
                n116 = VISA Write(VISA resource name=w707, write buffer=w712) -> (error out=w711:errorcluster)  [unwired: 1 in, 2 out]
                n117 = call <vilib>:"General Error Handler.vi"("error in (no error)"=w711) -> ()  [unwired: 10 in, 5 out]
              }
            }
          }
          event "电机失能": Value Change {
            n118 = event-data() -> ()  [unwired: 1 in, 6 out]
            n119 = property on="数值" class="DigNum (严格)"() -> ("Value"=w715:u8)  [unwired: 2 in, 2 out]
            n120 = case shown="真" "电机失能" {
              tunnel: w715 -> [_ w720]
              frame False {
              }
              frame True {
                n121 = Type Cast(x=w720) -> (*(type *) &x=w722:string)  [unwired: 1 in]
                n122 = Type Cast(x=u8 170) -> (*(type *) &x=w728:string)  [unwired: 1 in]
                n123 = Type Cast(x=u8 5) -> (*(type *) &x=w727:string)  [unwired: 1 in]
                n124 = Type Cast(x=u8 5) -> (*(type *) &x=w717:string)  [unwired: 1 in]
                n125 = Concatenate Strings(w728, w727, w722, w717, "/") -> (w726:string)
                n126 = property on="串口号" class="VISAName"() -> ("Value"=w721:refnum<visa-resource-name>)  [unwired: 2 in, 2 out]
                n127 = VISA Write(VISA resource name=w721, write buffer=w726) -> (error out=w725:errorcluster)  [unwired: 1 in, 2 out]
                n128 = call <vilib>:"General Error Handler.vi"("error in (no error)"=w725) -> ()  [unwired: 10 in, 5 out]
              }
            }
          }
          event "急停": Value Change {
            n129 = event-data() -> ()  [unwired: 1 in, 6 out]
            n130 = property on="数值" class="DigNum (严格)"() -> ("Value"=w729:u8)  [unwired: 2 in, 2 out]
            n131 = case shown="真" "急停" {
              tunnel: w729 -> [_ w735]
              frame False {
              }
              frame True {
                n132 = Type Cast(x=w735) -> (*(type *) &x=w736:string)  [unwired: 1 in]
                n133 = Type Cast(x=u8 170) -> (*(type *) &x=w742:string)  [unwired: 1 in]
                n134 = Type Cast(x=u8 6) -> (*(type *) &x=w741:string)  [unwired: 1 in]
                n135 = Type Cast(x=u8 5) -> (*(type *) &x=w731:string)  [unwired: 1 in]
                n136 = Concatenate Strings(w742, w741, w736, w731, "/") -> (w740:string)
                n137 = property on="串口号" class="VISAName"() -> ("Value"=w734:refnum<visa-resource-name>)  [unwired: 2 in, 2 out]
                n138 = VISA Write(VISA resource name=w734, write buffer=w740) -> (error out=w739:errorcluster)  [unwired: 1 in, 2 out]
                n139 = call <vilib>:"General Error Handler.vi"("error in (no error)"=w739) -> ()  [unwired: 10 in, 5 out]
              }
            }
          }
          event "示波器": Value Change {
            w761 = FALSE
            n140 = event-data() -> ()  [unwired: 1 in, 6 out]
            n141 = local read "参数1"() -> (w743:u8)
            n142 = local read "参数2"() -> (w758:T2)
            n143 = local read "参数3"() -> (w759:u8)
            n144 = local read "参数4"() -> (w744:u8)
            n145 = local write "电机2"(w761) -> ()
            n146 = local write "电机1"(w761) -> ()
            n147 = Type Cast(x=w743) -> (*(type *) &x=w753:string)  [unwired: 1 in]
            n148 = Type Cast(x=w758) -> (*(type *) &x=w754:string)  [unwired: 1 in]
            n149 = Type Cast(x=w759) -> (*(type *) &x=w755:string)  [unwired: 1 in]
            n150 = Type Cast(x=w744) -> (*(type *) &x=w756:string)  [unwired: 1 in]
            n151 = Type Cast(x=u8 170) -> (*(type *) &x=w751:string)  [unwired: 1 in]
            n152 = Type Cast(x=u8 27) -> (*(type *) &x=w752:string)  [unwired: 1 in]
            n153 = Type Cast(x=u8 8) -> (*(type *) &x=w757:string)  [unwired: 1 in]
            n154 = local write "参数监控"(w761) -> ()
            n155 = local write "运动控制"(w761) -> ()
            n156 = local write "串口设置"(w761) -> ()
            n157 = local write "选项卡控件"(T1."示波器" ("选项卡控件")) -> ()
            n158 = Concatenate Strings(w751, w752, w753, w754, w755, w756, w757, "/") -> (w749:string)
            n159 = property on="串口号" class="VISAName"() -> ("Value"=w760:refnum<visa-resource-name>)  [unwired: 2 in, 2 out]
            n160 = VISA Write(VISA resource name=w760, write buffer=w749) -> (error out=w750:errorcluster)  [unwired: 1 in, 2 out]
            n161 = call <vilib>:"General Error Handler.vi"("error in (no error)"=w750) -> ()  [unwired: 10 in, 5 out]
          }
          event "Flash保存": Value Change {
            n162 = event-data() -> ()  [unwired: 1 in, 6 out]
            n163 = Type Cast(x=u8 170) -> (*(type *) &x=w770:string)  [unwired: 1 in]
            n164 = Type Cast(x=u8 29) -> (*(type *) &x=w771:string)  [unwired: 1 in]
            n165 = Type Cast(x=u8 0) -> (*(type *) &x=w768:string)  [unwired: 1 in]
            n166 = Type Cast(x=u8 5) -> (*(type *) &x=w764:string)  [unwired: 1 in]
            n167 = Concatenate Strings(w770, w771, w768, w764, "/") -> (w772:string)
            n168 = property on="串口号" class="VISAName"() -> ("Value"=w766:refnum<visa-resource-name>)  [unwired: 2 in, 2 out]
            n169 = VISA Write(VISA resource name=w766, write buffer=w772) -> (error out=w773:errorcluster)  [unwired: 1 in, 2 out]
            n170 = call <vilib>:"General Error Handler.vi"("error in (no error)"=w773) -> ()  [unwired: 10 in, 5 out]
          }
          event "参数上传": Value Change {
            n171 = event-data() -> ()  [unwired: 1 in, 6 out]
            n172 = Type Cast(x=u8 170) -> (*(type *) &x=w783:string)  [unwired: 1 in]
            n173 = Type Cast(x=u8 30) -> (*(type *) &x=w782:string)  [unwired: 1 in]
            n174 = Type Cast(x=u8 0) -> (*(type *) &x=w784:string)  [unwired: 1 in]
            n175 = Type Cast(x=u8 5) -> (*(type *) &x=w786:string)  [unwired: 1 in]
            n176 = Concatenate Strings(w783, w782, w784, w786, "/") -> (w781:string)
            n177 = property on="串口号" class="VISAName"() -> ("Value"=w785:refnum<visa-resource-name>)  [unwired: 2 in, 2 out]
            n178 = VISA Write(VISA resource name=w785, write buffer=w781) -> (error out=w780:errorcluster)  [unwired: 1 in, 2 out]
            n179 = call <vilib>:"General Error Handler.vi"("error in (no error)"=w780) -> ()  [unwired: 10 in, 5 out]
          }
          event "写入3": Value Change {
            n180 = event-data() -> ()  [unwired: 1 in, 6 out]
            n181 = property on="ID" class="DigNum (严格)"("Value"="ID 3") -> ()  [unwired: 2 in, 2 out]
            n182 = property on="ID 2" class="DigNum (严格)"("Value"="ID 3") -> ()  [unwired: 2 in, 2 out]
            n183 = property on="数值1" class="DigNum (严格)"("Value"="数值3") -> ()  [unwired: 2 in, 2 out]
            n184 = property on="数值2" class="DigNum (严格)"("Value"="数值3") -> ()  [unwired: 2 in, 2 out]
            n185 = Type Cast(x="数值3") -> (*(type *) &x=w794:string)  [unwired: 1 in]
            n186 = Reverse String(1:w794) -> (0:w793:string)
            n187 = Type Cast(x="ID 3") -> (*(type *) &x=w795:string)  [unwired: 1 in]
            n188 = Type Cast(x=u8 170) -> (*(type *) &x=w799:string)  [unwired: 1 in]
            n189 = Type Cast(x=u8 10) -> (*(type *) &x=w798:string)  [unwired: 1 in]
            n190 = Type Cast(x=u8 10) -> (*(type *) &x=w792:string)  [unwired: 1 in]
            n191 = Type Cast(x=u8 1) -> (*(type *) &x=w800:string)  [unwired: 1 in]
            n192 = Concatenate Strings(w799, w798, w800, w795, w793, w792, "/") -> (w797:string)
            n193 = property on="串口号" class="VISAName"() -> ("Value"=w801:refnum<visa-resource-name>)  [unwired: 2 in, 2 out]
            n194 = VISA Write(VISA resource name=w801, write buffer=w797) -> (error out=w796:errorcluster)  [unwired: 1 in, 2 out]
            n195 = call <vilib>:"General Error Handler.vi"("error in (no error)"=w796) -> ()  [unwired: 10 in, 5 out]
          }
          event "读取 3": Value Change {
            n196 = event-data() -> ()  [unwired: 1 in, 6 out]
            n197 = property on="ID 3" class="DigNum (严格)"() -> ("Value"=w820:u8)  [unwired: 2 in, 2 out]
            n198 = property on="ID" class="DigNum (严格)"("Value"=w820) -> ()  [unwired: 2 in, 2 out]
            n199 = property on="ID 2" class="DigNum (严格)"("Value"=w820) -> ()  [unwired: 2 in, 2 out]
            n200 = Type Cast(x=0) -> (*(type *) &x=w812:string)  [unwired: 1 in]
            n201 = Reverse String(1:w812) -> (0:w811:string)
            n202 = Type Cast(x=w820) -> (*(type *) &x=w813:string)  [unwired: 1 in]
            n203 = Type Cast(x=u8 10) -> (*(type *) &x=w810:string)  [unwired: 1 in]
            n204 = Type Cast(x=u8 170) -> (*(type *) &x=w817:string)  [unwired: 1 in]
            n205 = Type Cast(x=u8 10) -> (*(type *) &x=w816:string)  [unwired: 1 in]
            n206 = Type Cast(x=u8 0) -> (*(type *) &x=w818:string)  [unwired: 1 in]
            n207 = Concatenate Strings(w817, w816, w818, w813, w811, w810, "/") -> (w815:string)
            n208 = property on="串口号" class="VISAName"() -> ("Value"=w819:refnum<visa-resource-name>)  [unwired: 2 in, 2 out]
            n209 = VISA Write(VISA resource name=w819, write buffer=w815) -> (error out=w814:errorcluster)  [unwired: 1 in, 2 out]
            n210 = call <vilib>:"General Error Handler.vi"("error in (no error)"=w814) -> ()  [unwired: 10 in, 5 out]
          }
          event "写入2": Value Change {
            n211 = event-data() -> ()  [unwired: 1 in, 6 out]
            n212 = property on="ID" class="DigNum (严格)"("Value"="ID 2") -> ()  [unwired: 2 in, 2 out]
            n213 = property on="ID 3" class="DigNum (严格)"("Value"="ID 2") -> ()  [unwired: 2 in, 2 out]
            n214 = property on="数值3" class="DigNum (严格)"("Value"="数值2") -> ()  [unwired: 2 in, 2 out]
            n215 = property on="数值1" class="DigNum (严格)"("Value"="数值2") -> ()  [unwired: 2 in, 2 out]
            n216 = Type Cast(x="数值2") -> (*(type *) &x=w828:string)  [unwired: 1 in]
            n217 = Reverse String(1:w828) -> (0:w827:string)
            n218 = Type Cast(x="ID 2") -> (*(type *) &x=w829:string)  [unwired: 1 in]
            n219 = Type Cast(x=u8 170) -> (*(type *) &x=w833:string)  [unwired: 1 in]
            n220 = Type Cast(x=u8 10) -> (*(type *) &x=w832:string)  [unwired: 1 in]
            n221 = Type Cast(x=u8 10) -> (*(type *) &x=w826:string)  [unwired: 1 in]
            n222 = Type Cast(x=u8 1) -> (*(type *) &x=w834:string)  [unwired: 1 in]
            n223 = Concatenate Strings(w833, w832, w834, w829, w827, w826, "/") -> (w831:string)
            n224 = property on="串口号" class="VISAName"() -> ("Value"=w835:refnum<visa-resource-name>)  [unwired: 2 in, 2 out]
            n225 = VISA Write(VISA resource name=w835, write buffer=w831) -> (error out=w830:errorcluster)  [unwired: 1 in, 2 out]
            n226 = call <vilib>:"General Error Handler.vi"("error in (no error)"=w830) -> ()  [unwired: 10 in, 5 out]
          }
          event "读取 2": Value Change {
            n227 = event-data() -> ()  [unwired: 1 in, 6 out]
            n228 = property on="ID 2" class="DigNum (严格)"() -> ("Value"=w854:u8)  [unwired: 2 in, 2 out]
            n229 = property on="ID 3" class="DigNum (严格)"("Value"=w854) -> ()  [unwired: 2 in, 2 out]
            n230 = property on="ID" class="DigNum (严格)"("Value"=w854) -> ()  [unwired: 2 in, 2 out]
            n231 = Type Cast(x=0) -> (*(type *) &x=w846:string)  [unwired: 1 in]
            n232 = Reverse String(1:w846) -> (0:w845:string)
            n233 = Type Cast(x=w854) -> (*(type *) &x=w847:string)  [unwired: 1 in]
            n234 = Type Cast(x=u8 10) -> (*(type *) &x=w844:string)  [unwired: 1 in]
            n235 = Type Cast(x=u8 170) -> (*(type *) &x=w851:string)  [unwired: 1 in]
            n236 = Type Cast(x=u8 10) -> (*(type *) &x=w850:string)  [unwired: 1 in]
            n237 = Type Cast(x=u8 0) -> (*(type *) &x=w852:string)  [unwired: 1 in]
            n238 = Concatenate Strings(w851, w850, w852, w847, w845, w844, "/") -> (w849:string)
            n239 = property on="串口号" class="VISAName"() -> ("Value"=w853:refnum<visa-resource-name>)  [unwired: 2 in, 2 out]
            n240 = VISA Write(VISA resource name=w853, write buffer=w849) -> (error out=w848:errorcluster)  [unwired: 1 in, 2 out]
            n241 = call <vilib>:"General Error Handler.vi"("error in (no error)"=w848) -> ()  [unwired: 10 in, 5 out]
          }
          event "写入": Value Change {
            n242 = event-data() -> ()  [unwired: 1 in, 6 out]
            n243 = property on="数值3" class="DigNum (严格)"("Value"="数值1") -> ()  [unwired: 2 in, 2 out]
            n244 = property on="数值2" class="DigNum (严格)"("Value"="数值1") -> ()  [unwired: 2 in, 2 out]
            n245 = property on="ID 2" class="DigNum (严格)"("Value"="ID") -> ()  [unwired: 2 in, 2 out]
            n246 = property on="ID 3" class="DigNum (严格)"("Value"="ID") -> ()  [unwired: 2 in, 2 out]
            n247 = Type Cast(x="数值1") -> (*(type *) &x=w863:string)  [unwired: 1 in]
            n248 = Reverse String(1:w863) -> (0:w862:string)
            n249 = Type Cast(x="ID") -> (*(type *) &x=w864:string)  [unwired: 1 in]
            n250 = Type Cast(x=u8 170) -> (*(type *) &x=w868:string)  [unwired: 1 in]
            n251 = Type Cast(x=u8 10) -> (*(type *) &x=w867:string)  [unwired: 1 in]
            n252 = Type Cast(x=u8 10) -> (*(type *) &x=w861:string)  [unwired: 1 in]
            n253 = Type Cast(x=u8 1) -> (*(type *) &x=w869:string)  [unwired: 1 in]
            n254 = Concatenate Strings(w868, w867, w869, w864, w862, w861, "/") -> (w866:string)
            n255 = property on="串口号" class="VISAName"() -> ("Value"=w870:refnum<visa-resource-name>)  [unwired: 2 in, 2 out]
            n256 = VISA Write(VISA resource name=w870, write buffer=w866) -> (error out=w865:errorcluster)  [unwired: 1 in, 2 out]
            n257 = call <vilib>:"General Error Handler.vi"("error in (no error)"=w865) -> ()  [unwired: 10 in, 5 out]
          }
          event "读取": Value Change {
            n258 = event-data() -> ()  [unwired: 1 in, 6 out]
            n259 = property on="ID" class="DigNum (严格)"() -> ("Value"=w888:u8)  [unwired: 2 in, 2 out]
            n260 = property on="ID 3" class="DigNum (严格)"("Value"=w888) -> ()  [unwired: 2 in, 2 out]
            n261 = property on="ID 2" class="DigNum (严格)"("Value"=w888) -> ()  [unwired: 2 in, 2 out]
            n262 = Type Cast(x=0) -> (*(type *) &x=w880:string)  [unwired: 1 in]
            n263 = Reverse String(1:w880) -> (0:w879:string)
            n264 = Type Cast(x=w888) -> (*(type *) &x=w881:string)  [unwired: 1 in]
            n265 = Type Cast(x=u8 10) -> (*(type *) &x=w878:string)  [unwired: 1 in]
            n266 = Type Cast(x=u8 170) -> (*(type *) &x=w885:string)  [unwired: 1 in]
            n267 = Type Cast(x=u8 10) -> (*(type *) &x=w884:string)  [unwired: 1 in]
            n268 = Type Cast(x=u8 0) -> (*(type *) &x=w886:string)  [unwired: 1 in]
            n269 = Concatenate Strings(w885, w884, w886, w881, w879, w878, "/") -> (w883:string)
            n270 = property on="串口号" class="VISAName"() -> ("Value"=w887:refnum<visa-resource-name>)  [unwired: 2 in, 2 out]
            n271 = VISA Write(VISA resource name=w887, write buffer=w883) -> (error out=w882:errorcluster)  [unwired: 1 in, 2 out]
            n272 = call <vilib>:"General Error Handler.vi"("error in (no error)"=w882) -> ()  [unwired: 10 in, 5 out]
          }
          event "清空显示": Value Change {
            n273 = event-data() -> ()  [unwired: 1 in, 6 out]
            n274 = property on="数      据      显      示" class="Str"("Value"="") -> ()  [unwired: 2 in, 2 out]
          }
          event "参数下发": Value Change {
            n275 = event-data() -> ()  [unwired: 1 in, 6 out]
            n276 = call "文件对话框"("prompt"="选择要读取的文件") -> ("selected path"=w892:path)  [unwired: 11 in, 3 out]
            n277 = Open/Create/Replace File(file path (use dialog)=w892) -> (refnum out=w893:refnum<file>, error out=w896:errorcluster)  [unwired: 5 in, 1 out]
            n278 = Set File Position(offset (in bytes) (0)=0, refnum=w893, error in=w896) -> (refnum out=w894:refnum<file>, error out=w898:errorcluster)  [unwired: 1 in]
            n279 = Read from Text File(file (use dialog)=w894, error in=w898) -> (refnum out=w895:refnum<file>, text=w901:string, error out=w897:errorcluster)  [unwired: 2 in, 1 out]
            "字符串" <- w901
            n280 = Close File(refnum=w895, error in=w897) -> ()  [unwired: 2 out]
            n281 = property on="串口号" class="VISAName"() -> ("Value"=w899:refnum<visa-resource-name>)  [unwired: 2 in, 2 out]
            n282 = VISA Write(VISA resource name=w899, write buffer=w901) -> (error out=w900:errorcluster)  [unwired: 1 in, 2 out]
            n283 = call <vilib>:"General Error Handler.vi"("error in (no error)"=w900) -> ()  [unwired: 10 in, 5 out]
          }
          event "保存数据": Value Change {
            n284 = event-data() -> ()  [unwired: 1 in, 6 out]
            n285 = property on="数      据      显      示" class="Str"() -> ("Value"=w902:string)  [unwired: 2 in, 2 out]
            n286 = call "文件对话框2"("prompt"="选择要存储的文件") -> ("selected path"=w907:path)  [unwired: 11 in, 3 out]
            n287 = Open/Create/Replace File(file path (use dialog)=w907, operation (0:open)=T3."open or create", access (0:read/write)=enum16{"read/write", "read-only", "write-only"}."read/write") -> (refnum out=w908:refnum<file>, error out=w910:errorcluster)  [unwired: 3 in, 1 out]
            n288 = Set File Position(offset (in bytes) (0)=0, refnum=w908, error in=w910) -> (refnum out=w909:refnum<file>, error out=w911:errorcluster)  [unwired: 1 in]
            n289 = Write to Text File(file (use dialog)=w909, text=w902, error in=w911) -> (refnum out=w912:refnum<file>, error out=w913:errorcluster)  [unwired: 1 in, 1 out]
            n290 = Close File(refnum=w912, error in=w913) -> ()  [unwired: 2 out]
          }
          event "发送电机参数": Value Change {
            n291 = event-data() -> ("OldVal"=w915:bool, "NewVal"=w916:bool)  [unwired: 1 in]
            n292 = Not(x=w915) -> (.not. x?=w917:bool)
            n293 = And(x=w917, y=w916) -> (x .and. y?=w914:bool)
            n294 = case shown="真" w914 {
              frame False {
              }
              frame True {
                # "发送电机1基本参数"
                n295 = property on="Pairs" class="DigNum (严格)"() -> ("Value"=w930:i32)  [unwired: 2 in, 2 out]
                n296 = property on="编码器分辨率" class="DigNum (严格)"() -> ("Value"=w924:u32)  [unwired: 2 in, 2 out]
                n297 = Type Cast(x=w930) -> (*(type *) &x=w932:string)  [unwired: 1 in]
                n298 = property on="力矩常数" class="DigNum (严格)"() -> ("Value"=w929:i32)  [unwired: 2 in, 2 out]
                n299 = property on="额定转速" class="DigNum (严格)"() -> ("Value"=w925:i32)  [unwired: 2 in, 2 out]
                n300 = property on="电机惯量" class="DigNum (严格)"() -> ("Value"=w928:i32)  [unwired: 2 in, 2 out]
                n301 = property on="额定电流" class="DigNum (严格)"() -> ("Value"=w927:i32)  [unwired: 2 in, 2 out]
                n302 = property on="额定转矩" class="DigNum (严格)"() -> ("Value"=w926:i32)  [unwired: 2 in, 2 out]
                n303 = Type Cast(x=w929) -> (*(type *) &x=w945:string)  [unwired: 1 in]
                n304 = Type Cast(x=w925) -> (*(type *) &x=w940:string)  [unwired: 1 in]
                n305 = Type Cast(x=w924) -> (*(type *) &x=w937:string)  [unwired: 1 in]
                n306 = Type Cast(x=w928) -> (*(type *) &x=w946:string)  [unwired: 1 in]
                n307 = Type Cast(x=w927) -> (*(type *) &x=w938:string)  [unwired: 1 in]
                n308 = Type Cast(x=w926) -> (*(type *) &x=w939:string)  [unwired: 1 in]
                n309 = Reverse String(1:w932) -> (0:w931:string)
                n310 = Reverse String(1:w945) -> (0:w948:string)
                n311 = Reverse String(1:w940) -> (0:w934:string)
                n312 = Reverse String(1:w937) -> (0:w933:string)
                n313 = Reverse String(1:w946) -> (0:w947:string)
                n314 = Reverse String(1:w938) -> (0:w936:string)
                n315 = Reverse String(1:w939) -> (0:w935:string)
                n316 = Type Cast(x=u8 17) -> (*(type *) &x=w942:string)  [unwired: 1 in]
                n317 = Type Cast(x=u8 32) -> (*(type *) &x=w918:string)  [unwired: 1 in]
                n318 = Type Cast(x=u8 170) -> (*(type *) &x=w941:string)  [unwired: 1 in]
                n319 = Concatenate Strings(w941, w942, w931, w948, w947, w936, w935, w934, w933, w918, "/") -> (w943:string)
                n320 = property on="串口号" class="VISAName"() -> ("Value"=w923:refnum<visa-resource-name>)  [unwired: 2 in, 2 out]
                n321 = VISA Write(VISA resource name=w923, write buffer=w943) -> (error out=w944:errorcluster)  [unwired: 1 in, 2 out]
                n322 = call <vilib>:"General Error Handler.vi"("error in (no error)"=w944) -> ()  [unwired: 10 in, 5 out]
              }
            }
          }
          event "发送电机参数 2": Value Change {
            n323 = event-data() -> ("OldVal"=w950:bool, "NewVal"=w951:bool)  [unwired: 1 in]
            n324 = Not(x=w950) -> (.not. x?=w952:bool)
            n325 = And(x=w952, y=w951) -> (x .and. y?=w949:bool)
            n326 = case shown="真" w949 {
              frame False {
              }
              frame True {
                # "发送电机2基本参数"
                n327 = Type Cast(x="Pairs 2") -> (*(type *) &x=w967:string)  [unwired: 1 in]
                n328 = Reverse String(1:w967) -> (0:w966:string)
                n329 = Type Cast(x="额定电流 2") -> (*(type *) &x=w973:string)  [unwired: 1 in]
                n330 = Type Cast(x="额定转矩 2") -> (*(type *) &x=w974:string)  [unwired: 1 in]
                n331 = Type Cast(x="额定转速 2") -> (*(type *) &x=w975:string)  [unwired: 1 in]
                n332 = Type Cast(x="编码器分辨率 2") -> (*(type *) &x=w972:string)  [unwired: 1 in]
                n333 = Reverse String(1:w972) -> (0:w968:string)
                n334 = Type Cast(x="力矩常数 2") -> (*(type *) &x=w980:string)  [unwired: 1 in]
                n335 = Type Cast(x="电机惯量 2") -> (*(type *) &x=w981:string)  [unwired: 1 in]
                n336 = Reverse String(1:w980) -> (0:w983:string)
                n337 = Reverse String(1:w981) -> (0:w982:string)
                n338 = Reverse String(1:w973) -> (0:w971:string)
                n339 = Reverse String(1:w974) -> (0:w970:string)
                n340 = Reverse String(1:w975) -> (0:w969:string)
                n341 = Type Cast(x=u8 20) -> (*(type *) &x=w977:string)  [unwired: 1 in]
                n342 = Type Cast(x=u8 170) -> (*(type *) &x=w976:string)  [unwired: 1 in]
                n343 = Type Cast(x=u8 32) -> (*(type *) &x=w954:string)  [unwired: 1 in]
                n344 = Concatenate Strings(w976, w977, w966, w983, w982, w971, w970, w969, w968, w954, "/") -> (w978:string)
                n345 = property on="串口号" class="VISAName"() -> ("Value"=w965:refnum<visa-resource-name>)  [unwired: 2 in, 2 out]
                n346 = VISA Write(VISA resource name=w965, write buffer=w978) -> (error out=w979:errorcluster)  [unwired: 1 in, 2 out]
                n347 = call <vilib>:"General Error Handler.vi"("error in (no error)"=w979) -> ()  [unwired: 10 in, 5 out]
              }
            }
          }
          event "发送保护参数": Value Change {
            n348 = event-data() -> ("OldVal"=w986:bool, "NewVal"=w985:bool)  [unwired: 1 in]
            n349 = Not(x=w986) -> (.not. x?=w987:bool)
            n350 = And(x=w987, y=w985) -> (x .and. y?=w984:bool)
            n351 = case shown="真" w984 {
              frame False {
              }
              frame True {
                # "发送电机1保护参数"
                n352 = property on="电机峰值电流" class="DigNum (严格)"() -> ("Value"=w997:i32)  [unwired: 2 in, 2 out]
                n353 = property on="最大相电流" class="DigNum (严格)"() -> ("Value"=w995:i32)  [unwired: 2 in, 2 out]
                n354 = property on="峰值电流持续时间" class="DigNum (严格)"() -> ("Value"=w996:i32)  [unwired: 2 in, 2 out]
                n355 = Type Cast(x=w997) -> (*(type *) &x=w1000:string)  [unwired: 1 in]
                n356 = Type Cast(x=w995) -> (*(type *) &x=w1016:string)  [unwired: 1 in]
                n357 = Reverse String(1:w1000) -> (0:w999:string)
                n358 = property on="最大速度" class="DigNum (严格)"() -> ("Value"=w994:i32)  [unwired: 2 in, 2 out]
                n359 = property on="堵转速度" class="DigNum (严格)"() -> ("Value"=w993:i32)  [unwired: 2 in, 2 out]
                n360 = property on="堵转电流" class="DigNum (严格)"() -> ("Value"=w992:i32)  [unwired: 2 in, 2 out]
                n361 = property on="堵转时间" class="DigNum (严格)"() -> ("Value"=w991:i32)  [unwired: 2 in, 2 out]
                n362 = Type Cast(x=w996) -> (*(type *) &x=w1015:string)  [unwired: 1 in]
                n363 = Type Cast(x=w994) -> (*(type *) &x=w1006:string)  [unwired: 1 in]
                n364 = Type Cast(x=w993) -> (*(type *) &x=w1007:string)  [unwired: 1 in]
                n365 = Type Cast(x=w992) -> (*(type *) &x=w1008:string)  [unwired: 1 in]
                n366 = Type Cast(x=w991) -> (*(type *) &x=w1005:string)  [unwired: 1 in]
                n367 = Reverse String(1:w1015) -> (0:w1018:string)
                n368 = Reverse String(1:w1016) -> (0:w1017:string)
                n369 = Reverse String(1:w1006) -> (0:w1004:string)
                n370 = Reverse String(1:w1007) -> (0:w1003:string)
                n371 = Reverse String(1:w1008) -> (0:w1002:string)
                n372 = Reverse String(1:w1005) -> (0:w1001:string)
                n373 = Type Cast(x=u8 18) -> (*(type *) &x=w1011:string)  [unwired: 1 in]
                n374 = Type Cast(x=u8 170) -> (*(type *) &x=w1010:string)  [unwired: 1 in]
                n375 = Type Cast(x=u8 32) -> (*(type *) &x=w989:string)  [unwired: 1 in]
                n376 = Concatenate Strings(w1010, w1011, w999, w1018, w1017, w1004, w1003, w1002, w1001, w989, "/") -> (w1012:string)
                n377 = property on="串口号" class="VISAName"() -> ("Value"=w998:refnum<visa-resource-name>)  [unwired: 2 in, 2 out]
                n378 = VISA Write(VISA resource name=w998, write buffer=w1012) -> (error out=w1013:errorcluster)  [unwired: 1 in, 2 out]
                n379 = call <vilib>:"General Error Handler.vi"("error in (no error)"=w1013) -> ()  [unwired: 10 in, 5 out]
              }
            }
          }
          event "发送保护参数 2": Value Change {
            n380 = event-data() -> ("OldVal"=w1021:bool, "NewVal"=w1020:bool)  [unwired: 1 in]
            n381 = Not(x=w1021) -> (.not. x?=w1022:bool)
            n382 = And(x=w1022, y=w1020) -> (x .and. y?=w1019:bool)
            n383 = case shown="真" w1019 {
              frame False {
              }
              frame True {
                # "发送电机2保护参数"
                n384 = Type Cast(x="电机峰值电流 2") -> (*(type *) &x=w1035:string)  [unwired: 1 in]
                n385 = Type Cast(x="最大相电流 2") -> (*(type *) &x=w1051:string)  [unwired: 1 in]
                n386 = Type Cast(x="最大速度 2") -> (*(type *) &x=w1041:string)  [unwired: 1 in]
                n387 = Type Cast(x="堵转速度 2") -> (*(type *) &x=w1042:string)  [unwired: 1 in]
                n388 = Type Cast(x="堵转电流 2") -> (*(type *) &x=w1043:string)  [unwired: 1 in]
                n389 = Type Cast(x="堵转时间 2") -> (*(type *) &x=w1040:string)  [unwired: 1 in]
                n390 = Reverse String(1:w1035) -> (0:w1034:string)
                n391 = Reverse String(1:w1041) -> (0:w1039:string)
                n392 = Reverse String(1:w1042) -> (0:w1038:string)
                n393 = Reverse String(1:w1043) -> (0:w1037:string)
                n394 = Reverse String(1:w1040) -> (0:w1036:string)
                n395 = Type Cast(x="峰值电流持续时间 2") -> (*(type *) &x=w1050:string)  [unwired: 1 in]
                n396 = Reverse String(1:w1050) -> (0:w1053:string)
                n397 = Reverse String(1:w1051) -> (0:w1052:string)
                n398 = Type Cast(x=u8 21) -> (*(type *) &x=w1046:string)  [unwired: 1 in]
                n399 = Type Cast(x=u8 170) -> (*(type *) &x=w1045:string)  [unwired: 1 in]
                n400 = Type Cast(x=u8 32) -> (*(type *) &x=w1024:string)  [unwired: 1 in]
                n401 = Concatenate Strings(w1045, w1046, w1034, w1053, w1052, w1039, w1038, w1037, w1036, w1024, "/") -> (w1047:string)
                n402 = property on="串口号" class="VISAName"() -> ("Value"=w1033:refnum<visa-resource-name>)  [unwired: 2 in, 2 out]
                n403 = VISA Write(VISA resource name=w1033, write buffer=w1047) -> (error out=w1048:errorcluster)  [unwired: 1 in, 2 out]
                n404 = call <vilib>:"General Error Handler.vi"("error in (no error)"=w1048) -> ()  [unwired: 10 in, 5 out]
              }
            }
          }
          event "发送 PID 1": Value Change {
            n405 = event-data() -> ("OldVal"=w1056:bool, "NewVal"=w1055:bool)  [unwired: 1 in]
            n406 = Not(x=w1056) -> (.not. x?=w1057:bool)
            n407 = And(x=w1057, y=w1055) -> (x .and. y?=w1054:bool)
            n408 = case shown="真" w1054 {
              frame False {
              }
              frame True {
                # "发送电机1PID参数"
                n409 = Type Cast(x="Pc1") -> (*(type *) &x=w1080:string)  [unwired: 1 in]
                n410 = Reverse String(1:w1080) -> (0:w1079:string)
                n411 = Type Cast(x="Ic 1") -> (*(type *) &x=w1096:string)  [unwired: 1 in]
                n412 = Type Cast(x="Pv1") -> (*(type *) &x=w1097:string)  [unwired: 1 in]
                n413 = Type Cast(x="Iv 1") -> (*(type *) &x=w1087:string)  [unwired: 1 in]
                n414 = Type Cast(x="Pp 1") -> (*(type *) &x=w1088:string)  [unwired: 1 in]
                n415 = Type Cast(x="Ip 1") -> (*(type *) &x=w1089:string)  [unwired: 1 in]
                n416 = Type Cast(x="Dp1") -> (*(type *) &x=w1086:string)  [unwired: 1 in]
                n417 = Type Cast(x="Ppll") -> (*(type *) &x=w1069:string)  [unwired: 1 in]
                n418 = Type Cast(x="Ipll") -> (*(type *) &x=w1068:string)  [unwired: 1 in]
                n419 = Type Cast(x="DIV1") -> (*(type *) &x=w1062:string)  [unwired: 1 in]
                n420 = Reverse String(1:w1096) -> (0:w1099:string)
                n421 = Reverse String(1:w1097) -> (0:w1098:string)
                n422 = Reverse String(1:w1087) -> (0:w1085:string)
                n423 = Reverse String(1:w1088) -> (0:w1084:string)
                n424 = Reverse String(1:w1089) -> (0:w1083:string)
                n425 = Reverse String(1:w1086) -> (0:w1082:string)
                n426 = Reverse String(1:w1069) -> (0:w1066:string)
                n427 = Reverse String(1:w1068) -> (0:w1064:string)
                n428 = Reverse String(1:w1062) -> (0:w1060:string)
                n429 = Type Cast(x="锁相环1") -> (*(type *) &x=w1070:string)  [unwired: 1 in]
                n430 = Type Cast(x=u8 19) -> (*(type *) &x=w1092:string)  [unwired: 1 in]
                n431 = Type Cast(x=u8 170) -> (*(type *) &x=w1091:string)  [unwired: 1 in]
                n432 = Type Cast(x=u8 45) -> (*(type *) &x=w1059:string)  [unwired: 1 in]
                n433 = Concatenate Strings(w1091, w1092, w1079, w1099, w1098, w1085, w1084, w1083, w1082, w1070, w1066, w1064, w1060, w1059, "/") -> (w1093:string)
                n434 = property on="串口号" class="VISAName"() -> ("Value"=w1081:refnum<visa-resource-name>)  [unwired: 2 in, 2 out]
                n435 = VISA Write(VISA resource name=w1081, write buffer=w1093) -> (error out=w1094:errorcluster)  [unwired: 1 in, 2 out]
                n436 = call <vilib>:"General Error Handler.vi"("error in (no error)"=w1094) -> ()  [unwired: 10 in, 5 out]
              }
            }
          }
          event "发送 PID 2": Value Change {
            n437 = event-data() -> ("OldVal"=w1102:bool, "NewVal"=w1101:bool)  [unwired: 1 in]
            n438 = Not(x=w1102) -> (.not. x?=w1103:bool)
            n439 = And(x=w1103, y=w1101) -> (x .and. y?=w1100:bool)
            n440 = case shown="真" w1100 {
              frame False {
              }
              frame True {
                # "发送电机2PID参数"
                n441 = Type Cast(x="Pc 2") -> (*(type *) &x=w1126:string)  [unwired: 1 in]
                n442 = Reverse String(1:w1126) -> (0:w1125:string)
                n443 = Type Cast(x="Ic2") -> (*(type *) &x=w1142:string)  [unwired: 1 in]
                n444 = Type Cast(x="Pv 2") -> (*(type *) &x=w1143:string)  [unwired: 1 in]
                n445 = Type Cast(x="Iv 2") -> (*(type *) &x=w1133:string)  [unwired: 1 in]
                n446 = Type Cast(x="Pp2") -> (*(type *) &x=w1134:string)  [unwired: 1 in]
                n447 = Type Cast(x="Ip 2") -> (*(type *) &x=w1135:string)  [unwired: 1 in]
                n448 = Type Cast(x="Dp2") -> (*(type *) &x=w1132:string)  [unwired: 1 in]
                n449 = Type Cast(x="Ppll 2") -> (*(type *) &x=w1115:string)  [unwired: 1 in]
                n450 = Type Cast(x="Ipll 2") -> (*(type *) &x=w1114:string)  [unwired: 1 in]
                n451 = Type Cast(x="DIV2") -> (*(type *) &x=w1108:string)  [unwired: 1 in]
                n452 = Reverse String(1:w1142) -> (0:w1145:string)
                n453 = Reverse String(1:w1143) -> (0:w1144:string)
                n454 = Reverse String(1:w1133) -> (0:w1131:string)
                n455 = Reverse String(1:w1134) -> (0:w1130:string)
                n456 = Reverse String(1:w1135) -> (0:w1129:string)
                n457 = Reverse String(1:w1132) -> (0:w1128:string)
                n458 = Reverse String(1:w1115) -> (0:w1112:string)
                n459 = Reverse String(1:w1114) -> (0:w1110:string)
                n460 = Reverse String(1:w1108) -> (0:w1105:string)
                n461 = Type Cast(x="锁相环2") -> (*(type *) &x=w1116:string)  [unwired: 1 in]
                n462 = Type Cast(x=u8 22) -> (*(type *) &x=w1138:string)  [unwired: 1 in]
                n463 = Type Cast(x=u8 170) -> (*(type *) &x=w1137:string)  [unwired: 1 in]
                n464 = Type Cast(x=u8 45) -> (*(type *) &x=w1104:string)  [unwired: 1 in]
                n465 = Concatenate Strings(w1137, w1138, w1125, w1145, w1144, w1131, w1130, w1129, w1128, w1116, w1112, w1110, w1105, w1104, "/") -> (w1139:string)
                n466 = property on="串口号" class="VISAName"() -> ("Value"=w1127:refnum<visa-resource-name>)  [unwired: 2 in, 2 out]
                n467 = VISA Write(VISA resource name=w1127, write buffer=w1139) -> (error out=w1140:errorcluster)  [unwired: 1 in, 2 out]
                n468 = call <vilib>:"General Error Handler.vi"("error in (no error)"=w1140) -> ()  [unwired: 10 in, 5 out]
              }
            }
          }
          event "运行模式": Value Change {
            n469 = event-data() -> ()  [unwired: 1 in, 6 out]
            n470 = control-ref of="运行模式"() -> (w1147:refnum<vi>)
            n471 = property class="TabCtl (严格)"(reference=w1147) -> ("Value"=w1146:enum32{"力矩模式", "速度模式", "位置模式"})  [unwired: 1 in, 2 out]
            "值" <- w1146
            n472 = case shown="\"力矩模式\"" w1146 {
              frame "位置模式", Default {
                n473 = property on="数值" class="DigNum (严格)"() -> ("Value"=w1152:u8)  [unwired: 2 in, 2 out]
                n474 = local write "数值 2"(3.0 ("数值 2")) -> ()
                n475 = Type Cast(x=w1152) -> (*(type *) &x=w1154:string)  [unwired: 1 in]
                n476 = Type Cast(x=u8 170) -> (*(type *) &x=w1156:string)  [unwired: 1 in]
                n477 = Type Cast(x=u8 13) -> (*(type *) &x=w1155:string)  [unwired: 1 in]
                n478 = Type Cast(x=u8 5) -> (*(type *) &x=w1149:string)  [unwired: 1 in]
                n479 = Concatenate Strings(w1156, w1155, w1154, w1149, "/") -> (w1158:string)
                n480 = property on="串口号" class="VISAName"() -> ("Value"=w1153:refnum<visa-resource-name>)  [unwired: 2 in, 2 out]
                n481 = VISA Write(VISA resource name=w1153, write buffer=w1158) -> (error out=w1157:errorcluster)  [unwired: 1 in, 2 out]
                n482 = call <vilib>:"General Error Handler.vi"("error in (no error)"=w1157) -> ()  [unwired: 10 in, 5 out]
              }
              frame "速度模式" {
                n483 = property on="数值" class="DigNum (严格)"() -> ("Value"=w1166:u8)  [unwired: 2 in, 2 out]
                n484 = local write "数值 2"(2.0 ("数值 2")) -> ()
                n485 = Type Cast(x=w1166) -> (*(type *) &x=w1167:string)  [unwired: 1 in]
                n486 = Type Cast(x=u8 170) -> (*(type *) &x=w1169:string)  [unwired: 1 in]
                n487 = Type Cast(x=u8 12) -> (*(type *) &x=w1168:string)  [unwired: 1 in]
                n488 = Type Cast(x=u8 5) -> (*(type *) &x=w1163:string)  [unwired: 1 in]
                n489 = Concatenate Strings(w1169, w1168, w1167, w1163, "/") -> (w1171:string)
                n490 = property on="串口号" class="VISAName"() -> ("Value"=w1165:refnum<visa-resource-name>)  [unwired: 2 in, 2 out]
                n491 = VISA Write(VISA resource name=w1165, write buffer=w1171) -> (error out=w1170:errorcluster)  [unwired: 1 in, 2 out]
                n492 = call <vilib>:"General Error Handler.vi"("error in (no error)"=w1170) -> ()  [unwired: 10 in, 5 out]
              }
              frame "力矩模式" {
                n493 = property on="数值" class="DigNum (严格)"() -> ("Value"=w1180:u8)  [unwired: 2 in, 2 out]
                n494 = local write "数值 2"(1.0 ("数值 2")) -> ()
                n495 = Type Cast(x=w1180) -> (*(type *) &x=w1179:string)  [unwired: 1 in]
                n496 = Type Cast(x=u8 170) -> (*(type *) &x=w1182:string)  [unwired: 1 in]
                n497 = Type Cast(x=u8 11) -> (*(type *) &x=w1181:string)  [unwired: 1 in]
                n498 = Type Cast(x=u8 5) -> (*(type *) &x=w1176:string)  [unwired: 1 in]
                n499 = Concatenate Strings(w1182, w1181, w1179, w1176, "/") -> (w1184:string)
                n500 = property on="串口号" class="VISAName"() -> ("Value"=w1178:refnum<visa-resource-name>)  [unwired: 2 in, 2 out]
                n501 = VISA Write(VISA resource name=w1178, write buffer=w1184) -> (error out=w1183:errorcluster)  [unwired: 1 in, 2 out]
                n502 = call <vilib>:"General Error Handler.vi"("error in (no error)"=w1183) -> ()  [unwired: 10 in, 5 out]
              }
            }
          }
          event "下发力矩参数": Value Change {
            n503 = event-data() -> ()  [unwired: 1 in, 4 out]
            n504 = Type Cast(x="目标力矩Motor 1") -> (*(type *) &x=w1197:string)  [unwired: 1 in]
            n505 = Type Cast(x="目标力矩Motor 2") -> (*(type *) &x=w1191:string)  [unwired: 1 in]
            n506 = property on="数值" class="DigNum (严格)"() -> ("Value"=w1194:u8)  [unwired: 2 in, 2 out]
            n507 = Reverse String(1:w1197) -> (0:w1195:string)
            n508 = Reverse String(1:w1191) -> (0:w1189:string)
            n509 = Type Cast(x=w1194) -> (*(type *) &x=w1198:string)  [unwired: 1 in]
            n510 = Type Cast(x=u8 170) -> (*(type *) &x=w1200:string)  [unwired: 1 in]
            n511 = Type Cast(x=u8 23) -> (*(type *) &x=w1199:string)  [unwired: 1 in]
            n512 = Type Cast(x=u8 13) -> (*(type *) &x=w1187:string)  [unwired: 1 in]
            n513 = Concatenate Strings(w1200, w1199, w1198, w1195, w1189, w1187, "/") -> (w1202:string)
            n514 = property on="串口号" class="VISAName"() -> ("Value"=w1193:refnum<visa-resource-name>)  [unwired: 2 in, 2 out]
            n515 = VISA Write(VISA resource name=w1193, write buffer=w1202) -> (error out=w1201:errorcluster)  [unwired: 1 in, 2 out]
            n516 = call <vilib>:"General Error Handler.vi"("error in (no error)"=w1201) -> ()  [unwired: 10 in, 5 out]
          }
          event "确认换向参数": Value Change {
            n517 = event-data() -> ()  [unwired: 1 in, 4 out]
            n518 = property on="数值" class="DigNum (严格)"() -> ("Value"=w1210:u8)  [unwired: 2 in, 2 out]
            n519 = Type Cast(x="换向电流") -> (*(type *) &x=w1212:string)  [unwired: 1 in]
            n520 = Reverse String(1:w1212) -> (0:w1211:string)
            n521 = Type Cast(x=w1210) -> (*(type *) &x=w1213:string)  [unwired: 1 in]
            n522 = Type Cast(x=u8 170) -> (*(type *) &x=w1215:string)  [unwired: 1 in]
            n523 = Type Cast(x=u8 9) -> (*(type *) &x=w1206:string)  [unwired: 1 in]
            n524 = Type Cast(x=u8 26) -> (*(type *) &x=w1214:string)  [unwired: 1 in]
            n525 = Concatenate Strings(w1215, w1214, w1213, w1211, w1206, "/") -> (w1217:string)
            n526 = property on="串口号" class="VISAName"() -> ("Value"=w1209:refnum<visa-resource-name>)  [unwired: 2 in, 2 out]
            n527 = VISA Write(VISA resource name=w1209, write buffer=w1217) -> (error out=w1216:errorcluster)  [unwired: 1 in, 2 out]
            n528 = call <vilib>:"General Error Handler.vi"("error in (no error)"=w1216) -> ()  [unwired: 10 in, 5 out]
          }
          event "下发速度参数": Value Change {
            n529 = event-data() -> ()  [unwired: 1 in, 6 out]
            n530 = Type Cast(x="目标速度Motor1") -> (*(type *) &x=w1236:string)  [unwired: 1 in]
            n531 = Type Cast(x="目标时间Motor1") -> (*(type *) &x=w1234:string)  [unwired: 1 in]
            n532 = Type Cast(x="目标速度Motor2") -> (*(type *) &x=w1227:string)  [unwired: 1 in]
            n533 = Type Cast(x="目标时间Motor2") -> (*(type *) &x=w1226:string)  [unwired: 1 in]
            n534 = property on="数值" class="DigNum (严格)"() -> ("Value"=w1232:u8)  [unwired: 2 in, 2 out]
            n535 = Reverse String(1:w1236) -> (0:w1235:string)
            n536 = Reverse String(1:w1234) -> (0:w1230:string)
            n537 = Reverse String(1:w1227) -> (0:w1224:string)
            n538 = Reverse String(1:w1226) -> (0:w1222:string)
            n539 = Type Cast(x=w1232) -> (*(type *) &x=w1237:string)  [unwired: 1 in]
            n540 = Type Cast(x=u8 170) -> (*(type *) &x=w1239:string)  [unwired: 1 in]
            n541 = Type Cast(x=u8 24) -> (*(type *) &x=w1238:string)  [unwired: 1 in]
            n542 = Type Cast(x=u8 21) -> (*(type *) &x=w1221:string)  [unwired: 1 in]
            n543 = Concatenate Strings(w1239, w1238, w1237, w1235, w1230, w1224, w1222, w1221, "/") -> (w1241:string)
            n544 = property on="串口号" class="VISAName"() -> ("Value"=w1233:refnum<visa-resource-name>)  [unwired: 2 in, 2 out]
            n545 = VISA Write(VISA resource name=w1233, write buffer=w1241) -> (error out=w1240:errorcluster)  [unwired: 1 in, 2 out]
            n546 = call <vilib>:"General Error Handler.vi"("error in (no error)"=w1240) -> ()  [unwired: 10 in, 5 out]
          }
          event "下发位置参数": Value Change {
            n547 = event-data() -> ()  [unwired: 1 in, 6 out]
            n548 = local read "目标速度 1"() -> (w1258:i32)
            n549 = local read "目标速度2"() -> (w1251:i32)
            n550 = Type Cast(x="目标位置Motor1") -> (*(type *) &x=w1272:string)  [unwired: 1 in]
            n551 = Type Cast(x=w1258) -> (*(type *) &x=w1270:string)  [unwired: 1 in]
            n552 = Type Cast(x="目标加速度Motor1") -> (*(type *) &x=w1269:string)  [unwired: 1 in]
            n553 = Type Cast(x="目标减速度Motor1") -> (*(type *) &x=w1263:string)  [unwired: 1 in]
            n554 = Type Cast(x="目标位置Motor2") -> (*(type *) &x=w1257:string)  [unwired: 1 in]
            n555 = Type Cast(x=w1251) -> (*(type *) &x=w1256:string)  [unwired: 1 in]
            n556 = Type Cast(x="目标加速度Motor2") -> (*(type *) &x=w1255:string)  [unwired: 1 in]
            n557 = Type Cast(x="目标减速度Motor2") -> (*(type *) &x=w1254:string)  [unwired: 1 in]
            n558 = property on="数值" class="DigNum (严格)"() -> ("Value"=w1265:u8)  [unwired: 2 in, 2 out]
            n559 = Reverse String(1:w1272) -> (0:w1271:string)
            n560 = Reverse String(1:w1270) -> (0:w1268:string)
            n561 = Reverse String(1:w1269) -> (0:w1267:string)
            n562 = Reverse String(1:w1263) -> (0:w1260:string)
            n563 = Reverse String(1:w1257) -> (0:w1252:string)
            n564 = Reverse String(1:w1256) -> (0:w1250:string)
            n565 = Reverse String(1:w1255) -> (0:w1248:string)
            n566 = Reverse String(1:w1254) -> (0:w1246:string)
            n567 = Type Cast(x=w1265) -> (*(type *) &x=w1273:string)  [unwired: 1 in]
            n568 = Type Cast(x=u8 170) -> (*(type *) &x=w1275:string)  [unwired: 1 in]
            n569 = Type Cast(x=u8 25) -> (*(type *) &x=w1274:string)  [unwired: 1 in]
            n570 = Type Cast(x=u8 37) -> (*(type *) &x=w1245:string)  [unwired: 1 in]
            n571 = Concatenate Strings(w1275, w1274, w1273, w1271, w1268, w1267, w1260, w1252, w1250, w1248, w1246, w1245, "/") -> (w1277:string)
            n572 = property on="串口号" class="VISAName"() -> ("Value"=w1266:refnum<visa-resource-name>)  [unwired: 2 in, 2 out]
            n573 = VISA Write(VISA resource name=w1266, write buffer=w1277) -> (error out=w1276:errorcluster)  [unwired: 1 in, 2 out]
            n574 = call <vilib>:"General Error Handler.vi"("error in (no error)"=w1276) -> ()  [unwired: 10 in, 5 out]
          }
          event "确认电机": Value Change {
            n575 = event-data() -> ()  [unwired: 1 in, 6 out]
            n576 = property on="数值" class="DigNum (严格)"() -> ("Value"=w1283:u8)  [unwired: 2 in, 2 out]
            n577 = local read "Motor1"() -> (w1295:bool)
            n578 = local read "Motor2"() -> (w1294:bool)
            n579 = Type Cast(x=w1283) -> (*(type *) &x=w1285:string)  [unwired: 1 in]
            n580 = Type Cast(x=u8 170) -> (*(type *) &x=w1287:string)  [unwired: 1 in]
            n581 = Type Cast(x=u8 14) -> (*(type *) &x=w1286:string)  [unwired: 1 in]
            n582 = Type Cast(x=u8 5) -> (*(type *) &x=w1281:string)  [unwired: 1 in]
            n583 = case shown="真" w1295 {
              tunnel: [u8 0 u8 1] -> w1292
              frame False {
              }
              frame True {
              }
            }
            n584 = case shown="真" w1294 {
              tunnel: [u8 0 u8 2] -> w1293
              frame False {
              }
              frame True {
              }
            }
            n585 = Concatenate Strings(w1287, w1286, w1285, w1281, "/") -> (w1289:string)
            n586 = property on="串口号" class="VISAName"() -> ("Value"=w1284:refnum<visa-resource-name>)  [unwired: 2 in, 2 out]
            n587 = VISA Write(VISA resource name=w1284, write buffer=w1289) -> (error out=w1288:errorcluster)  [unwired: 1 in, 2 out]
            n588 = call <vilib>:"General Error Handler.vi"("error in (no error)"=w1288) -> ()  [unwired: 10 in, 5 out]
            n589 = Add(x=w1292, y=w1293) -> (x+y=→"数值":u8)
          }
          event "确定运行模式": Value Change {
            n590 = event-data() -> ()  [unwired: 1 in, 6 out]
            n591 = property on="运行模式1" class="CmbBox"() -> ("Value"=w1305:string)  [unwired: 2 in, 2 out]
            n592 = case shown="\"3\"" w1305 {
              tunnel: [i8 4 i8 3 i8 1] -> w1301
              frame "1", Default {
              }
              frame "2" {
              }
              frame "3" {
              }
            }
            n593 = property on="数值" class="DigNum (严格)"() -> ("Value"=w1308:u8)  [unwired: 2 in, 2 out]
            n594 = Type Cast(x=w1308) -> (*(type *) &x=w1309:string)  [unwired: 1 in]
            n595 = Type Cast(x=w1301) -> (*(type *) &x=w1306:string)  [unwired: 1 in]
            n596 = Type Cast(x=u8 170) -> (*(type *) &x=w1311:string)  [unwired: 1 in]
            n597 = Type Cast(x=u8 8) -> (*(type *) &x=w1310:string)  [unwired: 1 in]
            n598 = Type Cast(x=u8 6) -> (*(type *) &x=w1302:string)  [unwired: 1 in]
            n599 = Concatenate Strings(w1311, w1310, w1309, w1306, w1302, "/") -> (w1313:string)
            n600 = property on="串口号" class="VISAName"() -> ("Value"=w1307:refnum<visa-resource-name>)  [unwired: 2 in, 2 out]
            n601 = VISA Write(VISA resource name=w1307, write buffer=w1313) -> (error out=w1312:errorcluster)  [unwired: 1 in, 2 out]
            n602 = call <vilib>:"General Error Handler.vi"("error in (no error)"=w1312) -> ()  [unwired: 10 in, 5 out]
          }
          event "位置取反": Value Change {
            n603 = event-data() -> ()  [unwired: 1 in, 6 out]
            n604 = local read "目标位置Motor1"() -> (w1330:i32)
            n605 = local read "目标位置Motor2"() -> (w1323:i32)
            n606 = Multiply(x="目标速度Motor1", y=1) -> (x*y=w1327:i32)
            n607 = Multiply(x="目标速度Motor2", y=1) -> (x*y=w1324:i32)
            n608 = Multiply(x=w1330, y=-1) -> (x*y=w1328:i32)
            n609 = Multiply(x=w1323, y=-1) -> (x*y=w1321:i32)
            n610 = local write "目标位置Motor1"(w1328) -> ()
            n611 = local write "目标位置Motor2"(w1321) -> ()
            n612 = local write "目标速度Motor1"(w1327) -> ()
            n613 = local write "目标速度Motor2"(w1324) -> ()
          }
          event "确认ID": Value Change {
            n614 = event-data() -> ()  [unwired: 1 in, 6 out]
            n615 = Type Cast(x="ID 1") -> (*(type *) &x=w1342:string)  [unwired: 1 in]
            n616 = Type Cast(x="ID 2") -> (*(type *) &x=w1340:string)  [unwired: 1 in]
            n617 = Type Cast(x="ID 3") -> (*(type *) &x=w1338:string)  [unwired: 1 in]
            n618 = Type Cast(x="ID 4") -> (*(type *) &x=w1337:string)  [unwired: 1 in]
            n619 = Type Cast(x=u8 170) -> (*(type *) &x=w1344:string)  [unwired: 1 in]
            n620 = Type Cast(x=u8 28) -> (*(type *) &x=w1343:string)  [unwired: 1 in]
            n621 = Type Cast(x=u8 8) -> (*(type *) &x=w1336:string)  [unwired: 1 in]
            n622 = Concatenate Strings(w1344, w1343, w1342, w1340, w1338, w1337, w1336, "/") -> (w1346:string)
            n623 = property on="串口号" class="VISAName"() -> ("Value"=w1341:refnum<visa-resource-name>)  [unwired: 2 in, 2 out]
            n624 = VISA Write(VISA resource name=w1341, write buffer=w1346) -> (error out=w1345:errorcluster)  [unwired: 1 in, 2 out]
            n625 = call <vilib>:"General Error Handler.vi"("error in (no error)"=w1345) -> ()  [unwired: 10 in, 5 out]
          }
          event "参数确定": Value Change {
            n626 = event-data() -> ()  [unwired: 1 in, 6 out]
            n627 = Type Cast(x="参数1") -> (*(type *) &x=w1360:string)  [unwired: 1 in]
            n628 = Type Cast(x="参数2") -> (*(type *) &x=w1358:string)  [unwired: 1 in]
            n629 = Type Cast(x="参数3") -> (*(type *) &x=w1356:string)  [unwired: 1 in]
            n630 = Type Cast(x="参数4") -> (*(type *) &x=w1355:string)  [unwired: 1 in]
            n631 = Type Cast(x=u8 170) -> (*(type *) &x=w1362:string)  [unwired: 1 in]
            n632 = Type Cast(x=u8 27) -> (*(type *) &x=w1361:string)  [unwired: 1 in]
            n633 = Type Cast(x=u8 8) -> (*(type *) &x=w1354:string)  [unwired: 1 in]
            n634 = Concatenate Strings(w1362, w1361, w1360, w1358, w1356, w1355, w1354, "/") -> (w1364:string)
            n635 = property on="串口号" class="VISAName"() -> ("Value"=w1359:refnum<visa-resource-name>)  [unwired: 2 in, 2 out]
            n636 = VISA Write(VISA resource name=w1359, write buffer=w1364) -> (error out=w1363:errorcluster)  [unwired: 1 in, 2 out]
            n637 = call <vilib>:"General Error Handler.vi"("error in (no error)"=w1363) -> ()  [unwired: 10 in, 5 out]
          }
          event "同步模式开关": Value Change {
            n638 = event-data() -> ()  [unwired: 1 in, 6 out]
            n639 = case shown="假" "同步模式开关" {
              frame False {
                n640 = Type Cast(x=u8 170) -> (*(type *) &x=w1379:string)  [unwired: 1 in]
                n641 = Type Cast(x=u8 15) -> (*(type *) &x=w1378:string)  [unwired: 1 in]
                n642 = Type Cast(x=u8 1) -> (*(type *) &x=w1373:string)  [unwired: 1 in]
                n643 = Type Cast(x=u8 5) -> (*(type *) &x=w1369:string)  [unwired: 1 in]
                n644 = Concatenate Strings(w1379, w1378, w1373, w1369, "/") -> (w1377:string)
                n645 = property on="串口号" class="VISAName"() -> ("Value"=w1372:refnum<visa-resource-name>)  [unwired: 2 in, 2 out]
                n646 = VISA Write(VISA resource name=w1372, write buffer=w1377) -> (error out=w1376:errorcluster)  [unwired: 1 in, 2 out]
                n647 = call <vilib>:"General Error Handler.vi"("error in (no error)"=w1376) -> ()  [unwired: 10 in, 5 out]
              }
              frame True {
                n648 = Type Cast(x=u8 170) -> (*(type *) &x=w1391:string)  [unwired: 1 in]
                n649 = Type Cast(x=u8 15) -> (*(type *) &x=w1390:string)  [unwired: 1 in]
                n650 = Type Cast(x=u8 0) -> (*(type *) &x=w1385:string)  [unwired: 1 in]
                n651 = Type Cast(x=u8 5) -> (*(type *) &x=w1381:string)  [unwired: 1 in]
                n652 = Concatenate Strings(w1391, w1390, w1385, w1381, "/") -> (w1389:string)
                n653 = property on="串口号" class="VISAName"() -> ("Value"=w1384:refnum<visa-resource-name>)  [unwired: 2 in, 2 out]
                n654 = VISA Write(VISA resource name=w1384, write buffer=w1389) -> (error out=w1388:errorcluster)  [unwired: 1 in, 2 out]
                n655 = call <vilib>:"General Error Handler.vi"("error in (no error)"=w1388) -> ()  [unwired: 10 in, 5 out]
              }
            }
          }
        }
        n656 = case shown="假" "弧度脉冲" {
          frame False {
            w45 = 1
            n657 = local read "目标速度Motor2"() -> (w44:i32)
            n658 = Divide(x=1, y=w45) -> (x/y=w48:dbl)
            n659 = Multiply(x=w44, y=w48) -> (x*y=w47:dbl)
            n660 = Multiply(x=w47, y=w45) -> (x*y=w43:dbl)
            n661 = local write "目标速度2"(w43) -> ()
          }
          frame True {
            n662 = local read "目标速度Motor2"() -> (w50:i32)
            n663 = Divide(x=100, y=6.283185307179586) -> (x/y=w55:dbl)
            n664 = Multiply(x=w50, y=w55) -> (x*y=w54:dbl)
            n665 = Multiply(x=w54, y=1) -> (x*y=→"目标速度2":dbl)
          }
        }
        n666 = case shown="假" "弧度脉冲" {
          frame False {
            w57 = 1
            n667 = local read "目标速度Motor1"() -> (w62:i32)
            n668 = Divide(x=1, y=w57) -> (x/y=w61:dbl)
            n669 = Multiply(x=w62, y=w61) -> (x*y=w60:dbl)
            n670 = Multiply(x=w60, y=w57) -> (x*y=w59:dbl)
            n671 = local write "目标速度 1"(w59) -> ()
          }
          frame True {
            n672 = local read "目标速度Motor1"() -> (w69:i32)
            n673 = Divide(x=100, y=6.283185307179586) -> (x/y=w68:dbl)
            n674 = Multiply(x=w69, y=w68) -> (x*y=w67:dbl)
            n675 = Multiply(x=w67, y=1) -> (x*y=→"目标速度 1":dbl)
          }
        }
        n676 = property on="数      据      显      示" class="Str"() -> ("Value"=w33:string)  [unwired: 2 in, 2 out]
        n677 = VISA Read(VISA resource name=w34, byte count=w41) -> (VISA resource name out=w19:refnum<visa-resource-name>, read buffer=w25:string)  [unwired: 1 in, 2 out]
        n678 = String To Byte Array(string=w25) -> (unsigned byte array=w24:u8[])
        "无符号字节数组" <- w24
        n679 = Concatenate Strings(w33, w25) -> (w29:string)
        "数      据      显      示" <- w29
        n680 = Array Size(array=w24) -> (size(s)=w21:i32)
        "数值 5" <- w21
        n681 = Index Array(array=w24, index=0) -> (element=w39:u8)
        n682 = String Length(string=w29) -> (length=w32:i32)
        n683 = Equal?(x=w39, y=u8 170) -> (x = y?=w27:bool)
        n684 = Decrement(x=w21) -> (x-1=w36:i32)
        n685 = Greater?(x=w32, y=2000) -> (0:w30:bool)
        n686 = Index Array(array=w24, index=w36) -> (element=w22:u8)
        n687 = case shown="真" w30 {
          frame False {
          }
          frame True {
            n688 = property on="数      据      显      示" class="Str"("Value"="") -> ()  [unwired: 2 in, 2 out]
          }
        }
        n689 = Equal?(x=w22, y=u8 47) -> (x = y?=w26:bool)
        n690 = Compound Arithmetic op=AND ("复合运算")(w27, w26) -> (w23:bool)
        n691 = case shown="真" w23 {
          tunnel: w24 -> [_ w77]
          tunnel: w22 -> [_ w72]
          frame False {
            n692 = local write "布尔"(TRUE ("布尔")) -> ()
            n693 = Wait Until Next ms Multiple(millisecond multiple=u32 1 ("毫秒倍数")) -> ()  [unwired: 1 out]
          }
          frame True {
            # "提取指令码"
            n694 = local read "数值 3"() -> (w74:dbl)
            n695 = Index Array(array=w77, index=1) -> (element=w78:u8)
            n696 = case shown="88" w78 {
              tunnel: w77 -> [w84 w109 w227 w399 w426 w486 w500 w515 w557 w570 _]
              frame 128 {
                n697 = Not(x="停止") -> (.not. x?=w81:bool)
                n698 = And(x=TRUE, y=w81) -> (x .and. y?=w80:bool)
                n699 = case shown="真" w80 {
                  tunnel: w84 -> [_ w85]
                  frame False {
                  }
                  frame True {
                    w98 = 0
                    w96 = 0
                    # "指令码是0x80"
                    n700 = Array Subset(array=w85, index=2, length=4) -> (w107:u8[])
                    n701 = Array Subset(array=w85, index=6, length=4) -> (w93:u8[])
                    n702 = Array Subset(array=w85, index=10, length=4) -> (w92:u8[])
                    n703 = Array Subset(array=w85, index=14, length=4) -> (w91:u8[])
                    n704 = Reverse 1D Array(array=w107) -> (reversed array=w105:u8[])
                    n705 = Reverse 1D Array(array=w93) -> (reversed array=w97:u8[])
                    n706 = Type Cast(type=w96, x=w97) -> (*(type *) &x=w89:i32)
                    n707 = Reverse 1D Array(array=w92) -> (reversed array=w95:u8[])
                    n708 = Reverse 1D Array(array=w91) -> (reversed array=w94:u8[])
                    n709 = Type Cast(type=w96, x=w105) -> (*(type *) &x=w90:i32)
                    n710 = Type Cast(type=w98, x=w95) -> (*(type *) &x=w88:i32)
                    n711 = Type Cast(type=w98, x=w94) -> (*(type *) &x=w87:i32)
                    n712 = Bundle(w90, w89, w88, w87) -> (→"波形图表":cluster{i32, i32, i32, i32})  [unwired: 1 in]
                  }
                }
              }
              frame 129 {
                w129 = 4
                w131 = u32 0
                w175 = 0
                w173 = 4
                w197 = 0
                w198 = 4
                # "电机1参数反馈"
                # "指令码是0x81"
                n713 = Array Subset(array=w109, index=82, length=4) -> (w154:u8[])
                n714 = Array Subset(array=w109, index=86, length=1) -> (w139:u8[])
                n715 = Array Subset(array=w109, index=87, length=4) -> (w144:u8[])
                n716 = Array Subset(array=w109, index=58, length=4) -> (w166:u8[])
                n717 = Array Subset(array=w109, index=62, length=4) -> (w164:u8[])
                n718 = Array Subset(array=w109, index=66, length=4) -> (w162:u8[])
                n719 = Array Subset(array=w109, index=70, length=4) -> (w160:u8[])
                n720 = Array Subset(array=w109, index=74, length=4) -> (w158:u8[])
                n721 = Array Subset(array=w109, index=78, length=4) -> (w156:u8[])
                n722 = Array Subset(array=w109, index=2, length=w198) -> (w225:u8[])
                n723 = Array Subset(array=w109, index=6, length=w198) -> (w222:u8[])
                n724 = Array Subset(array=w109, index=22, length=w198) -> (w210:u8[])
                n725 = Array Subset(array=w109, index=26, length=w198) -> (w207:u8[])
                n726 = Array Subset(array=w109, index=30, length=w173) -> (w196:u8[])
                n727 = Array Subset(array=w109, index=34, length=w173) -> (w194:u8[])
                n728 = Array Subset(array=w109, index=38, length=w173) -> (w192:u8[])
                n729 = Array Subset(array=w109, index=42, length=w173) -> (w190:u8[])
                n730 = Array Subset(array=w109, index=10, length=w198) -> (w219:u8[])
                n731 = Array Subset(array=w109, index=14, length=w198) -> (w216:u8[])
                n732 = Array Subset(array=w109, index=18, length=w198) -> (w213:u8[])
                n733 = Array Subset(array=w109, index=46, length=w173) -> (w188:u8[])
                n734 = Array Subset(array=w109, index=50, length=w173) -> (w186:u8[])
                n735 = Array Subset(array=w109, index=54, length=w173) -> (w184:u8[])
                n736 = Array Subset(array=w109, index=91, length=w129) -> (w143:u8[])
                n737 = Array Subset(array=w109, index=95, length=w129) -> (w134:u8[])
                n738 = Reverse 1D Array(array=w225) -> (reversed array=w224:u8[])
                n739 = Reverse 1D Array(array=w222) -> (reversed array=w221:u8[])
                n740 = Reverse 1D Array(array=w210) -> (reversed array=w209:u8[])
                n741 = Reverse 1D Array(array=w207) -> (reversed array=w206:u8[])
                n742 = Reverse 1D Array(array=w196) -> (reversed array=w195:u8[])
                n743 = Reverse 1D Array(array=w194) -> (reversed array=w193:u8[])
                n744 = Reverse 1D Array(array=w192) -> (reversed array=w191:u8[])
                n745 = Reverse 1D Array(array=w190) -> (reversed array=w189:u8[])
                n746 = Reverse 1D Array(array=w219) -> (reversed array=w218:u8[])
                n747 = Reverse 1D Array(array=w216) -> (reversed array=w215:u8[])
                n748 = Reverse 1D Array(array=w213) -> (reversed array=w212:u8[])
                n749 = Reverse 1D Array(array=w188) -> (reversed array=w187:u8[])
                n750 = Reverse 1D Array(array=w186) -> (reversed array=w185:u8[])
                n751 = Reverse 1D Array(array=w184) -> (reversed array=w183:u8[])
                n752 = Reverse 1D Array(array=w143) -> (reversed array=w142:u8[])
                n753 = Reverse 1D Array(array=w134) -> (reversed array=w133:u8[])
                n754 = Reverse 1D Array(array=w154) -> (reversed array=w153:u8[])
                n755 = Reverse 1D Array(array=w139) -> (reversed array=w138:u8[])
                n756 = Reverse 1D Array(array=w144) -> (reversed array=w145:u8[])
                n757 = Reverse 1D Array(array=w166) -> (reversed array=w165:u8[])
                n758 = Reverse 1D Array(array=w164) -> (reversed array=w163:u8[])
                n759 = Reverse 1D Array(array=w162) -> (reversed array=w161:u8[])
                n760 = Reverse 1D Array(array=w160) -> (reversed array=w159:u8[])
                n761 = Reverse 1D Array(array=w158) -> (reversed array=w157:u8[])
                n762 = Reverse 1D Array(array=w156) -> (reversed array=w155:u8[])
                n763 = Type Cast(type=w197, x=w224) -> (*(type *) &x=w205:i32)
                n764 = Type Cast(type=w197, x=w221) -> (*(type *) &x=w204:i32)
                n765 = Type Cast(type=w197, x=w209) -> (*(type *) &x=w201:i32)
                n766 = Type Cast(type=w197, x=w206) -> (*(type *) &x=w200:i32)
                n767 = Type Cast(type=w175, x=w195) -> (*(type *) &x=w182:i32)
                n768 = Type Cast(type=w175, x=w193) -> (*(type *) &x=w176:i32)
                n769 = Type Cast(type=w175, x=w191) -> (*(type *) &x=w181:i32)
                n770 = Type Cast(type=w175, x=w189) -> (*(type *) &x=w178:i32)
                n771 = Type Cast(type=w197, x=w218) -> (*(type *) &x=w199:i32)
                n772 = Type Cast(type=w197, x=w215) -> (*(type *) &x=w203:i32)
                n773 = Type Cast(type=w197, x=w212) -> (*(type *) &x=w202:i32)
                n774 = Type Cast(type=w175, x=w187) -> (*(type *) &x=w177:i32)
                n775 = Type Cast(type=w175, x=w185) -> (*(type *) &x=w180:i32)
                n776 = Type Cast(type=w175, x=w183) -> (*(type *) &x=w179:i32)
                n777 = Type Cast(type=w131, x=w142) -> (*(type *) &x=w140:u32)
                n778 = Type Cast(type=w131, x=w133) -> (*(type *) &x=w132:u32)
                n779 = Type Cast(type=w131, x=w153) -> (*(type *) &x=w147:u32)
                n780 = Type Cast(type=w131, x=w138) -> (*(type *) &x=w137:u32)
                n781 = Type Cast(type=w131, x=w145) -> (*(type *) &x=w141:u32)
                n782 = Type Cast(type=w131, x=w165) -> (*(type *) &x=w146:u32)
                n783 = Type Cast(type=w131, x=w163) -> (*(type *) &x=w152:u32)
                n784 = Type Cast(type=w131, x=w161) -> (*(type *) &x=w151:u32)
                n785 = Type Cast(type=w131, x=w159) -> (*(type *) &x=w150:u32)
                n786 = Type Cast(type=w131, x=w157) -> (*(type *) &x=w149:u32)
                n787 = Type Cast(type=w131, x=w155) -> (*(type *) &x=w148:u32)
                n788 = property on="Pairs" class="DigNum (严格)"("Value"=w205) -> ()  [unwired: 2 in, 2 out]
                n789 = property on="力矩常数" class="DigNum (严格)"("Value"=w204) -> ()  [unwired: 2 in, 2 out]
                n790 = property on="额定转速" class="DigNum (严格)"("Value"=w201) -> ()  [unwired: 2 in, 2 out]
                n791 = property on="编码器分辨率" class="DigNum (严格)"("Value"=w200) -> ()  [unwired: 2 in, 2 out]
                n792 = property on="电机峰值电流" class="DigNum (严格)"("Value"=w182) -> ()  [unwired: 2 in, 2 out]
                n793 = property on="峰值电流持续时间" class="DigNum (严格)"("Value"=w176) -> ()  [unwired: 2 in, 2 out]
                n794 = property on="最大相电流" class="DigNum (严格)"("Value"=w181) -> ()  [unwired: 2 in, 2 out]
                n795 = property on="最大速度" class="DigNum (严格)"("Value"=w178) -> ()  [unwired: 2 in, 2 out]
                n796 = property on="电机惯量" class="DigNum (严格)"("Value"=w199) -> ()  [unwired: 2 in, 2 out]
                n797 = property on="额定电流" class="DigNum (严格)"("Value"=w203) -> ()  [unwired: 2 in, 2 out]
                n798 = property on="额定转矩" class="DigNum (严格)"("Value"=w202) -> ()  [unwired: 2 in, 2 out]
                n799 = property on="堵转速度" class="DigNum (严格)"("Value"=w177) -> ()  [unwired: 2 in, 2 out]
                n800 = property on="堵转电流" class="DigNum (严格)"("Value"=w180) -> ()  [unwired: 2 in, 2 out]
                n801 = property on="堵转时间" class="DigNum (严格)"("Value"=w179) -> ()  [unwired: 2 in, 2 out]
                n802 = property on="Ipll" class="DigNum (严格)"("Value"=w140) -> ()  [unwired: 2 in, 2 out]
                n803 = property on="DIV1" class="DigNum (严格)"("Value"=w132) -> ()  [unwired: 2 in, 2 out]
                n804 = property on="Dp1" class="DigNum (严格)"("Value"=w147) -> ()  [unwired: 2 in, 2 out]
                n805 = property on="Ppll" class="DigNum (严格)"("Value"=w141) -> ()  [unwired: 2 in, 2 out]
                n806 = property on="Pc1" class="DigNum (严格)"("Value"=w146) -> ()  [unwired: 2 in, 2 out]
                n807 = property on="Ic 1" class="DigNum (严格)"("Value"=w152) -> ()  [unwired: 2 in, 2 out]
                n808 = property on="Pv1" class="DigNum (严格)"("Value"=w151) -> ()  [unwired: 2 in, 2 out]
                n809 = property on="Iv 1" class="DigNum (严格)"("Value"=w150) -> ()  [unwired: 2 in, 2 out]
                n810 = property on="Pp 1" class="DigNum (严格)"("Value"=w149) -> ()  [unwired: 2 in, 2 out]
                n811 = property on="Ip 1" class="DigNum (严格)"("Value"=w148) -> ()  [unwired: 2 in, 2 out]
                n812 = Number To Boolean Array(number=w137) -> (Boolean array=w136:bool[])
                n813 = Or Array Elements(Boolean array=w136) -> (logical OR=w135:bool)
                n814 = property on="锁相环1" class="Bool (严格)"("Value"=w135) -> ()  [unwired: 2 in, 2 out]
              }
              frame 132 {
                w290 = 4
                w292 = u32 0
                w270 = 0
                w228 = 4
                w262 = 0
                w260 = 4
                # "电机2参数反馈"
                # "指令码是0x84"
                n815 = Array Subset(array=w227, index=82, length=4) -> (w304:u8[])
                n816 = Array Subset(array=w227, index=86, length=1) -> (w298:u8[])
                n817 = Array Subset(array=w227, index=87, length=4) -> (w301:u8[])
                n818 = Array Subset(array=w227, index=58, length=4) -> (w316:u8[])
                n819 = Array Subset(array=w227, index=62, length=4) -> (w314:u8[])
                n820 = Array Subset(array=w227, index=66, length=4) -> (w312:u8[])
                n821 = Array Subset(array=w227, index=70, length=4) -> (w310:u8[])
                n822 = Array Subset(array=w227, index=74, length=4) -> (w308:u8[])
                n823 = Array Subset(array=w227, index=78, length=4) -> (w306:u8[])
                n824 = Array Subset(array=w227, index=91, length=w290) -> (w300:u8[])
                n825 = Array Subset(array=w227, index=10, length=w260) -> (w340:u8[])
                n826 = Array Subset(array=w227, index=14, length=w260) -> (w338:u8[])
                n827 = Array Subset(array=w227, index=2, length=w260) -> (w344:u8[])
                n828 = Array Subset(array=w227, index=6, length=w260) -> (w342:u8[])
                n829 = Array Subset(array=w227, index=30, length=w228) -> (w330:u8[])
                n830 = Array Subset(array=w227, index=34, length=w228) -> (w328:u8[])
                n831 = Array Subset(array=w227, index=38, length=w228) -> (w326:u8[])
                n832 = Array Subset(array=w227, index=54, length=w228) -> (w318:u8[])
                n833 = Array Subset(array=w227, index=18, length=w260) -> (w336:u8[])
                n834 = Array Subset(array=w227, index=22, length=w260) -> (w334:u8[])
                n835 = Array Subset(array=w227, index=26, length=w260) -> (w332:u8[])
                n836 = Array Subset(array=w227, index=42, length=w228) -> (w324:u8[])
                n837 = Array Subset(array=w227, index=46, length=w228) -> (w322:u8[])
                n838 = Array Subset(array=w227, index=50, length=w228) -> (w320:u8[])
                n839 = Array Subset(array=w227, index=95, length=w290) -> (w294:u8[])
                n840 = Reverse 1D Array(array=w304) -> (reversed array=w303:u8[])
                n841 = Reverse 1D Array(array=w298) -> (reversed array=w297:u8[])
                n842 = Reverse 1D Array(array=w301) -> (reversed array=w302:u8[])
                n843 = Reverse 1D Array(array=w300) -> (reversed array=w299:u8[])
                n844 = Reverse 1D Array(array=w340) -> (reversed array=w339:u8[])
                n845 = Reverse 1D Array(array=w338) -> (reversed array=w337:u8[])
                n846 = Reverse 1D Array(array=w342) -> (reversed array=w341:u8[])
                n847 = Reverse 1D Array(array=w330) -> (reversed array=w329:u8[])
                n848 = Reverse 1D Array(array=w328) -> (reversed array=w327:u8[])
                n849 = Reverse 1D Array(array=w326) -> (reversed array=w325:u8[])
                n850 = Reverse 1D Array(array=w318) -> (reversed array=w317:u8[])
                n851 = Reverse 1D Array(array=w336) -> (reversed array=w335:u8[])
                n852 = Reverse 1D Array(array=w334) -> (reversed array=w333:u8[])
                n853 = Reverse 1D Array(array=w332) -> (reversed array=w331:u8[])
                n854 = Reverse 1D Array(array=w324) -> (reversed array=w323:u8[])
                n855 = Reverse 1D Array(array=w322) -> (reversed array=w321:u8[])
                n856 = Reverse 1D Array(array=w320) -> (reversed array=w319:u8[])
                n857 = Reverse 1D Array(array=w294) -> (reversed array=w293:u8[])
                n858 = Reverse 1D Array(array=w316) -> (reversed array=w315:u8[])
                n859 = Reverse 1D Array(array=w314) -> (reversed array=w313:u8[])
                n860 = Reverse 1D Array(array=w312) -> (reversed array=w311:u8[])
                n861 = Reverse 1D Array(array=w310) -> (reversed array=w309:u8[])
                n862 = Reverse 1D Array(array=w308) -> (reversed array=w307:u8[])
                n863 = Reverse 1D Array(array=w306) -> (reversed array=w305:u8[])
                n864 = Type Cast(type=w292, x=w303) -> (*(type *) &x=w233:u32)
                n865 = Type Cast(type=w292, x=w297) -> (*(type *) &x=w296:u32)
                n866 = Type Cast(type=w292, x=w302) -> (*(type *) &x=w231:u32)
                n867 = Type Cast(type=w292, x=w299) -> (*(type *) &x=w230:u32)
                n868 = Type Cast(type=w262, x=w339) -> (*(type *) &x=w251:i32)
                n869 = Type Cast(type=w262, x=w337) -> (*(type *) &x=w250:i32)
                n870 = Type Cast(type=w262, x=w341) -> (*(type *) &x=w252:i32)
                n871 = Type Cast(type=w270, x=w329) -> (*(type *) &x=w246:i32)
                n872 = Type Cast(type=w270, x=w327) -> (*(type *) &x=w245:i32)
                n873 = Type Cast(type=w270, x=w325) -> (*(type *) &x=w244:i32)
                n874 = Type Cast(type=w270, x=w317) -> (*(type *) &x=w240:i32)
                n875 = Type Cast(type=w262, x=w335) -> (*(type *) &x=w249:i32)
                n876 = Type Cast(type=w262, x=w333) -> (*(type *) &x=w248:i32)
                n877 = Type Cast(type=w262, x=w331) -> (*(type *) &x=w247:i32)
                n878 = Type Cast(type=w270, x=w323) -> (*(type *) &x=w243:i32)
                n879 = Type Cast(type=w270, x=w321) -> (*(type *) &x=w242:i32)
                n880 = Type Cast(type=w270, x=w319) -> (*(type *) &x=w241:i32)
                n881 = Type Cast(type=w292, x=w293) -> (*(type *) &x=w229:u32)
                n882 = Type Cast(type=w292, x=w315) -> (*(type *) &x=w239:u32)
                n883 = Type Cast(type=w292, x=w313) -> (*(type *) &x=w238:u32)
                n884 = Type Cast(type=w292, x=w311) -> (*(type *) &x=w237:u32)
                n885 = Type Cast(type=w292, x=w309) -> (*(type *) &x=w236:u32)
                n886 = Type Cast(type=w292, x=w307) -> (*(type *) &x=w235:u32)
                n887 = Type Cast(type=w292, x=w305) -> (*(type *) &x=w234:u32)
                n888 = property on="Dp2" class="DigNum (严格)"("Value"=w233) -> ()  [unwired: 2 in, 2 out]
                n889 = property on="Ppll 2" class="DigNum (严格)"("Value"=w231) -> ()  [unwired: 2 in, 2 out]
                n890 = property on="Ipll 2" class="DigNum (严格)"("Value"=w230) -> ()  [unwired: 2 in, 2 out]
                n891 = property on="电机惯量 2" class="DigNum (严格)"("Value"=w251) -> ()  [unwired: 2 in, 2 out]
                n892 = property on="额定电流 2" class="DigNum (严格)"("Value"=w250) -> ()  [unwired: 2 in, 2 out]
                n893 = property on="力矩常数 2" class="DigNum (严格)"("Value"=w252) -> ()  [unwired: 2 in, 2 out]
                n894 = property on="电机峰值电流 2" class="DigNum (严格)"("Value"=w246) -> ()  [unwired: 2 in, 2 out]
                n895 = property on="峰值电流持续时间 2" class="DigNum (严格)"("Value"=w245) -> ()  [unwired: 2 in, 2 out]
                n896 = property on="最大相电流 2" class="DigNum (严格)"("Value"=w244) -> ()  [unwired: 2 in, 2 out]
                n897 = property on="堵转时间 2" class="DigNum (严格)"("Value"=w240) -> ()  [unwired: 2 in, 2 out]
                n898 = property on="额定转矩 2" class="DigNum (严格)"("Value"=w249) -> ()  [unwired: 2 in, 2 out]
                n899 = property on="额定转速 2" class="DigNum (严格)"("Value"=w248) -> ()  [unwired: 2 in, 2 out]
                n900 = property on="编码器分辨率 2" class="DigNum (严格)"("Value"=w247) -> ()  [unwired: 2 in, 2 out]
                n901 = property on="最大速度 2" class="DigNum (严格)"("Value"=w243) -> ()  [unwired: 2 in, 2 out]
                n902 = property on="堵转速度 2" class="DigNum (严格)"("Value"=w242) -> ()  [unwired: 2 in, 2 out]
                n903 = property on="堵转电流 2" class="DigNum (严格)"("Value"=w241) -> ()  [unwired: 2 in, 2 out]
                n904 = property on="DIV2" class="DigNum (严格)"("Value"=w229) -> ()  [unwired: 2 in, 2 out]
                n905 = property on="Pc 2" class="DigNum (严格)"("Value"=w239) -> ()  [unwired: 2 in, 2 out]
                n906 = property on="Ic2" class="DigNum (严格)"("Value"=w238) -> ()  [unwired: 2 in, 2 out]
                n907 = property on="Pv 2" class="DigNum (严格)"("Value"=w237) -> ()  [unwired: 2 in, 2 out]
                n908 = property on="Iv 2" class="DigNum (严格)"("Value"=w236) -> ()  [unwired: 2 in, 2 out]
                n909 = property on="Pp2" class="DigNum (严格)"("Value"=w235) -> ()  [unwired: 2 in, 2 out]
                n910 = property on="Ip 2" class="DigNum (严格)"("Value"=w234) -> ()  [unwired: 2 in, 2 out]
                n911 = Number To Boolean Array(number=w296) -> (Boolean array=w295:bool[])
                n912 = Or Array Elements(Boolean array=w295) -> (logical OR=w232:bool)
                n913 = property on="锁相环2" class="Bool (严格)"("Value"=w232) -> ()  [unwired: 2 in, 2 out]
                n914 = Reverse 1D Array(array=w344) -> (reversed array=w343:u8[])
                n915 = Type Cast(type=w262, x=w343) -> (*(type *) &x=w253:i32)
                n916 = property on="Pairs 2" class="DigNum (严格)"("Value"=w253) -> ()  [unwired: 2 in, 2 out]
              }
              frame 133 {
                w397 = 2
                # "电机2保护参数反馈"
                # "指令码是0x85"
                n917 = Array Subset(array=w399, index=4, length=w397) -> (w348:u8[])
                n918 = Array Subset(array=w399, index=2, length=w397) -> (w350:u8[])
                n919 = Array Subset(array=w399, index=8, length=w397) -> (w396:u8[])
                n920 = Array Subset(array=w399, index=6, length=w397) -> (w421:u8[])
                n921 = Array Subset(array=w399, index=12, length=w397) -> (w395:u8[])
                n922 = Array Subset(array=w399, index=10, length=w397) -> (w419:u8[])
                n923 = Array Subset(array=w399, index=16, length=w397) -> (w394:u8[])
                n924 = Array Subset(array=w399, index=14, length=w397) -> (w416:u8[])
                n925 = Array Subset(array=w399, index=20, length=w397) -> (w393:u8[])
                n926 = Array Subset(array=w399, index=18, length=w397) -> (w413:u8[])
                n927 = Array Subset(array=w399, index=24, length=w397) -> (w392:u8[])
                n928 = Array Subset(array=w399, index=22, length=w397) -> (w410:u8[])
                n929 = Array Subset(array=w399, index=28, length=w397) -> (w391:u8[])
                n930 = Array Subset(array=w399, index=26, length=w397) -> (w407:u8[])
                n931 = Reverse 1D Array(array=w350) -> (reversed array=w349:u8[])
                n932 = Reverse 1D Array(array=w348) -> (reversed array=w347:u8[])
                n933 = Reverse 1D Array(array=w396) -> (reversed array=w386:u8[])
                n934 = Reverse 1D Array(array=w421) -> (reversed array=w387:u8[])
                n935 = Reverse 1D Array(array=w395) -> (reversed array=w385:u8[])
                n936 = Reverse 1D Array(array=w419) -> (reversed array=w418:u8[])
                n937 = Reverse 1D Array(array=w394) -> (reversed array=w384:u8[])
                n938 = Reverse 1D Array(array=w416) -> (reversed array=w415:u8[])
                n939 = Reverse 1D Array(array=w393) -> (reversed array=w383:u8[])
                n940 = Reverse 1D Array(array=w413) -> (reversed array=w412:u8[])
                n941 = Reverse 1D Array(array=w392) -> (reversed array=w382:u8[])
                n942 = Reverse 1D Array(array=w410) -> (reversed array=w409:u8[])
                n943 = Reverse 1D Array(array=w391) -> (reversed array=w381:u8[])
                n944 = Reverse 1D Array(array=w407) -> (reversed array=w406:u8[])
                n945 = Type Cast(x=w386) -> (*(type *) &x=w373:string)  [unwired: 1 in]
                n946 = Type Cast(x=w387) -> (*(type *) &x=w374:string)  [unwired: 1 in]
                n947 = Type Cast(x=w385) -> (*(type *) &x=w369:string)  [unwired: 1 in]
                n948 = Type Cast(x=w418) -> (*(type *) &x=w370:string)  [unwired: 1 in]
                n949 = Type Cast(x=w384) -> (*(type *) &x=w365:string)  [unwired: 1 in]
                n950 = Type Cast(x=w415) -> (*(type *) &x=w366:string)  [unwired: 1 in]
                n951 = Type Cast(x=w383) -> (*(type *) &x=w361:string)  [unwired: 1 in]
                n952 = Type Cast(x=w412) -> (*(type *) &x=w362:string)  [unwired: 1 in]
                n953 = Type Cast(x=w382) -> (*(type *) &x=w357:string)  [unwired: 1 in]
                n954 = Type Cast(x=w409) -> (*(type *) &x=w358:string)  [unwired: 1 in]
                n955 = Type Cast(x=w381) -> (*(type *) &x=w353:string)  [unwired: 1 in]
                n956 = Type Cast(x=w406) -> (*(type *) &x=w354:string)  [unwired: 1 in]
                n957 = Concatenate Strings(w373, w374) -> (w372:string)
                n958 = Concatenate Strings(w369, w370) -> (w368:string)
                n959 = Concatenate Strings(w365, w366) -> (w364:string)
                n960 = Concatenate Strings(w361, w362) -> (w360:string)
                n961 = Concatenate Strings(w357, w358) -> (w356:string)
                n962 = Concatenate Strings(w353, w354) -> (w352:string)
                n963 = Type Cast(x=w347) -> (*(type *) &x=w345:string)  [unwired: 1 in]
                n964 = Type Cast(x=w349) -> (*(type *) &x=w346:string)  [unwired: 1 in]
                n965 = Concatenate Strings(w345, w346) -> (w389:string)
                n966 = Type Cast(type=0, x=w372) -> (*(type *) &x=w371:i32)
                n967 = Type Cast(type=0, x=w368) -> (*(type *) &x=w367:i32)
                n968 = Type Cast(type=0, x=w364) -> (*(type *) &x=w363:i32)
                n969 = Type Cast(type=0, x=w360) -> (*(type *) &x=w359:i32)
                n970 = Type Cast(type=0, x=w356) -> (*(type *) &x=w355:i32)
                n971 = Type Cast(type=0, x=w352) -> (*(type *) &x=w351:i32)
                n972 = property on="峰值电流持续时间 2" class="DigNum (严格)"("Value"=w371) -> ()  [unwired: 2 in, 2 out]
                n973 = property on="最大相电流 2" class="DigNum (严格)"("Value"=w367) -> ()  [unwired: 2 in, 2 out]
                n974 = property on="最大速度 2" class="DigNum (严格)"("Value"=w363) -> ()  [unwired: 2 in, 2 out]
                n975 = property on="堵转速度 2" class="DigNum (严格)"("Value"=w359) -> ()  [unwired: 2 in, 2 out]
                n976 = property on="堵转电流 2" class="DigNum (严格)"("Value"=w355) -> ()  [unwired: 2 in, 2 out]
                n977 = property on="堵转时间 2" class="DigNum (严格)"("Value"=w351) -> ()  [unwired: 2 in, 2 out]
                n978 = Type Cast(type=0, x=w389) -> (*(type *) &x=w388:i32)
                n979 = property on="电机峰值电流 2" class="DigNum (严格)"("Value"=w388) -> ()  [unwired: 2 in, 2 out]
              }
              frame 134 {
                w424 = u32 0
                # "PID参数反馈2"
                # "指令码是0x86"
                n980 = Array Subset(array=w426, index=2, length=4) -> (w481:u8[])
                n981 = Array Subset(array=w426, index=6, length=4) -> (w477:u8[])
                n982 = Array Subset(array=w426, index=10, length=4) -> (w474:u8[])
                n983 = Array Subset(array=w426, index=26, length=4) -> (w462:u8[])
                n984 = Array Subset(array=w426, index=30, length=1) -> (w437:u8[])
                n985 = Array Subset(array=w426, index=31, length=4) -> (w446:u8[])
                n986 = Array Subset(array=w426, index=14, length=4) -> (w471:u8[])
                n987 = Array Subset(array=w426, index=18, length=4) -> (w468:u8[])
                n988 = Array Subset(array=w426, index=22, length=4) -> (w465:u8[])
                n989 = Array Subset(array=w426, index=35, length=4) -> (w445:u8[])
                n990 = Array Subset(array=w426, index=39, length=4) -> (w430:u8[])
                n991 = Reverse 1D Array(array=w481) -> (reversed array=w479:u8[])
                n992 = Reverse 1D Array(array=w477) -> (reversed array=w476:u8[])
                n993 = Type Cast(type=w424, x=w479) -> (*(type *) &x=w454:u32)
                n994 = Type Cast(type=w424, x=w476) -> (*(type *) &x=w453:u32)
                n995 = Reverse 1D Array(array=w474) -> (reversed array=w473:u8[])
                n996 = Reverse 1D Array(array=w462) -> (reversed array=w461:u8[])
                n997 = Reverse 1D Array(array=w437) -> (reversed array=w436:u8[])
                n998 = Reverse 1D Array(array=w446) -> (reversed array=w447:u8[])
                n999 = Reverse 1D Array(array=w471) -> (reversed array=w470:u8[])
                n1000 = Reverse 1D Array(array=w468) -> (reversed array=w467:u8[])
                n1001 = Reverse 1D Array(array=w465) -> (reversed array=w464:u8[])
                n1002 = Reverse 1D Array(array=w445) -> (reversed array=w444:u8[])
                n1003 = Reverse 1D Array(array=w430) -> (reversed array=w429:u8[])
                n1004 = property on="Pc 2" class="DigNum (严格)"("Value"=w454) -> ()  [unwired: 2 in, 2 out]
                n1005 = property on="Ic2" class="DigNum (严格)"("Value"=w453) -> ()  [unwired: 2 in, 2 out]
                n1006 = Type Cast(type=w424, x=w473) -> (*(type *) &x=w452:u32)
                n1007 = Type Cast(type=w424, x=w461) -> (*(type *) &x=w448:u32)
                n1008 = Type Cast(type=w424, x=w436) -> (*(type *) &x=w435:u32)
                n1009 = Type Cast(type=w424, x=w447) -> (*(type *) &x=w432:u32)
                n1010 = Type Cast(type=w424, x=w470) -> (*(type *) &x=w451:u32)
                n1011 = Type Cast(type=w424, x=w467) -> (*(type *) &x=w450:u32)
                n1012 = Type Cast(type=w424, x=w464) -> (*(type *) &x=w449:u32)
                n1013 = Type Cast(type=w424, x=w444) -> (*(type *) &x=w431:u32)
                n1014 = Type Cast(type=w424, x=w429) -> (*(type *) &x=w425:u32)
                n1015 = property on="Pv 2" class="DigNum (严格)"("Value"=w452) -> ()  [unwired: 2 in, 2 out]
                n1016 = property on="Dp2" class="DigNum (严格)"("Value"=w448) -> ()  [unwired: 2 in, 2 out]
                n1017 = property on="Ppll 2" class="DigNum (严格)"("Value"=w432) -> ()  [unwired: 2 in, 2 out]
                n1018 = property on="Iv 2" class="DigNum (严格)"("Value"=w451) -> ()  [unwired: 2 in, 2 out]
                n1019 = property on="Pp2" class="DigNum (严格)"("Value"=w450) -> ()  [unwired: 2 in, 2 out]
                n1020 = property on="Ip 2" class="DigNum (严格)"("Value"=w449) -> ()  [unwired: 2 in, 2 out]
                n1021 = property on="Ipll 2" class="DigNum (严格)"("Value"=w431) -> ()  [unwired: 2 in, 2 out]
                n1022 = property on="DIV2" class="DigNum (严格)"("Value"=w425) -> ()  [unwired: 2 in, 2 out]
                n1023 = Number To Boolean Array(number=w435) -> (Boolean array=w434:bool[])
                n1024 = Or Array Elements(Boolean array=w434) -> (logical OR=w433:bool)
                n1025 = property on="锁相环2" class="Bool (严格)"("Value"=w433) -> ()  [unwired: 2 in, 2 out]
              }
              frame 135 {
                w485 = 4
                # "电机1参数反馈"
                # "指令码是0x81"
                n1026 = Array Subset(array=w486, index=2, length=w485) -> (w493:u8[])
                n1027 = Array Subset(array=w486, index=6, length=w485) -> (w489:u8[])
                n1028 = Reverse 1D Array(array=w493) -> (reversed array=w492:u8[])
                n1029 = Reverse 1D Array(array=w489) -> (reversed array=w488:u8[])
                n1030 = Type Cast(type=0, x=w492) -> (*(type *) &x=w490:i32)
                n1031 = Type Cast(type=0, x=w488) -> (*(type *) &x=w484:i32)
                n1032 = property on="目标力矩Motor 1" class="DigNum (严格)"("Value"=w490) -> ()  [unwired: 2 in, 2 out]
                n1033 = property on="目标力矩Motor 2" class="DigNum (严格)"("Value"=w484) -> ()  [unwired: 2 in, 2 out]
              }
              frame 136 {
                w501 = 0
                w508 = 0
                w499 = 4
                n1034 = Array Subset(array=w500, index=2, length=w499) -> (w513:u8[])
                n1035 = Array Subset(array=w500, index=6, length=w499) -> (w510:u8[])
                n1036 = Array Subset(array=w500, index=10, length=w499) -> (w505:u8[])
                n1037 = Array Subset(array=w500, index=14, length=w499) -> (w503:u8[])
                n1038 = Reverse 1D Array(array=w513) -> (reversed array=w512:u8[])
                n1039 = Reverse 1D Array(array=w510) -> (reversed array=w509:u8[])
                n1040 = Reverse 1D Array(array=w505) -> (reversed array=w504:u8[])
                n1041 = Reverse 1D Array(array=w503) -> (reversed array=w502:u8[])
                n1042 = Type Cast(type=w508, x=w512) -> (*(type *) &x=w507:i32)
                n1043 = Type Cast(type=w508, x=w509) -> (*(type *) &x=w506:i32)
                n1044 = Type Cast(type=w501, x=w504) -> (*(type *) &x=w498:i32)
                n1045 = Type Cast(type=w501, x=w502) -> (*(type *) &x=w497:i32)
                n1046 = property on="目标速度Motor1" class="DigNum (严格)"("Value"=w507) -> ()  [unwired: 2 in, 2 out]
                n1047 = property on="目标时间Motor1" class="DigNum (严格)"("Value"=w506) -> ()  [unwired: 2 in, 2 out]
                n1048 = property on="目标速度Motor2" class="DigNum (严格)"("Value"=w498) -> ()  [unwired: 2 in, 2 out]
                n1049 = property on="目标时间Motor2" class="DigNum (严格)"("Value"=w497) -> ()  [unwired: 2 in, 2 out]
              }
              frame 137 {
                w521 = 0
                w520 = 4
                w529 = 0
                w528 = 4
                w541 = 0
                w540 = 4
                w549 = 0
                w548 = 4
                n1050 = Array Subset(array=w515, index=2, length=w548) -> (w554:u8[])
                n1051 = Array Subset(array=w515, index=6, length=w548) -> (w551:u8[])
                n1052 = Array Subset(array=w515, index=10, length=w540) -> (w546:u8[])
                n1053 = Array Subset(array=w515, index=14, length=w540) -> (w543:u8[])
                n1054 = Array Subset(array=w515, index=18, length=w528) -> (w534:u8[])
                n1055 = Array Subset(array=w515, index=22, length=w528) -> (w531:u8[])
                n1056 = Array Subset(array=w515, index=26, length=w520) -> (w526:u8[])
                n1057 = Array Subset(array=w515, index=30, length=w520) -> (w523:u8[])
                n1058 = Reverse 1D Array(array=w554) -> (reversed array=w553:u8[])
                n1059 = Reverse 1D Array(array=w551) -> (reversed array=w550:u8[])
                n1060 = Reverse 1D Array(array=w546) -> (reversed array=w545:u8[])
                n1061 = Reverse 1D Array(array=w543) -> (reversed array=w542:u8[])
                n1062 = Reverse 1D Array(array=w534) -> (reversed array=w533:u8[])
                n1063 = Reverse 1D Array(array=w531) -> (reversed array=w530:u8[])
                n1064 = Reverse 1D Array(array=w526) -> (reversed array=w525:u8[])
                n1065 = Reverse 1D Array(array=w523) -> (reversed array=w522:u8[])
                n1066 = Type Cast(type=w549, x=w553) -> (*(type *) &x=w536:i32)
                n1067 = Type Cast(type=w549, x=w550) -> (*(type *) &x=w537:i32)
                n1068 = Type Cast(type=w541, x=w545) -> (*(type *) &x=w538:i32)
                n1069 = Type Cast(type=w541, x=w542) -> (*(type *) &x=w539:i32)
                n1070 = Type Cast(type=w529, x=w533) -> (*(type *) &x=w519:i32)
                n1071 = Type Cast(type=w529, x=w530) -> (*(type *) &x=w518:i32)
                n1072 = Type Cast(type=w521, x=w525) -> (*(type *) &x=w517:i32)
                n1073 = Type Cast(type=w521, x=w522) -> (*(type *) &x=w516:i32)
                n1074 = property on="目标位置Motor1" class="DigNum (严格)"("Value"=w536) -> ()  [unwired: 2 in, 2 out]
                n1075 = property on="目标速度Motor1" class="DigNum (严格)"("Value"=w537) -> ()  [unwired: 2 in, 2 out]
                n1076 = property on="目标加速度Motor1" class="DigNum (严格)"("Value"=w538) -> ()  [unwired: 2 in, 2 out]
                n1077 = property on="目标减速度Motor1" class="DigNum (严格)"("Value"=w539) -> ()  [unwired: 2 in, 2 out]
                n1078 = property on="目标位置Motor2" class="DigNum (严格)"("Value"=w519) -> ()  [unwired: 2 in, 2 out]
                n1079 = property on="目标速度Motor2" class="DigNum (严格)"("Value"=w518) -> ()  [unwired: 2 in, 2 out]
                n1080 = property on="目标加速度Motor2" class="DigNum (严格)"("Value"=w517) -> ()  [unwired: 2 in, 2 out]
                n1081 = property on="目标减速度Motor2" class="DigNum (严格)"("Value"=w516) -> ()  [unwired: 2 in, 2 out]
              }
              frame 138 {
                n1082 = Array Subset(array=w557, index=2, length=4) -> (w561:u8[])
                n1083 = Reverse 1D Array(array=w561) -> (reversed array=w560:u8[])
                n1084 = Type Cast(type=0, x=w560) -> (*(type *) &x=w556:i32)
                "数值1 2" <- w556
                n1085 = property on="数值1" class="DigNum (严格)"("Value"=w556) -> ()  [unwired: 2 in, 2 out]
                n1086 = property on="数值2" class="DigNum (严格)"("Value"=w556) -> ()  [unwired: 2 in, 2 out]
                n1087 = property on="数值3" class="DigNum (严格)"("Value"=w556) -> ()  [unwired: 2 in, 2 out]
              }
              frame 144 {
                w568 = 0
                w569 = 4
                # "监控参数反馈"
                # "指令码是0x90"
                n1088 = Array Subset(array=w570, index=2, length=w569) -> (w608:u8[])
                n1089 = Array Subset(array=w570, index=6, length=w569) -> (w605:u8[])
                n1090 = Array Subset(array=w570, index=10, length=w569) -> (w602:u8[])
                n1091 = Array Subset(array=w570, index=14, length=w569) -> (w599:u8[])
                n1092 = Array Subset(array=w570, index=18, length=w569) -> (w596:u8[])
                n1093 = Array Subset(array=w570, index=22, length=w569) -> (w593:u8[])
                n1094 = Array Subset(array=w570, index=26, length=w569) -> (w590:u8[])
                n1095 = Array Subset(array=w570, index=30, length=w569) -> (w575:u8[])
                n1096 = Array Subset(array=w570, index=34, length=w569) -> (w576:u8[])
                n1097 = Array Subset(array=w570, index=38, length=w569) -> (w574:u8[])
                n1098 = Array Subset(array=w570, index=42, length=w569) -> (w571:u8[])
                n1099 = Reverse 1D Array(array=w608) -> (reversed array=w607:u8[])
                n1100 = Reverse 1D Array(array=w605) -> (reversed array=w604:u8[])
                n1101 = Reverse 1D Array(array=w602) -> (reversed array=w601:u8[])
                n1102 = Reverse 1D Array(array=w599) -> (reversed array=w598:u8[])
                n1103 = Reverse 1D Array(array=w596) -> (reversed array=w595:u8[])
                n1104 = Reverse 1D Array(array=w593) -> (reversed array=w592:u8[])
                n1105 = Reverse 1D Array(array=w590) -> (reversed array=w589:u8[])
                n1106 = Reverse 1D Array(array=w575) -> (reversed array=w577:u8[])
                n1107 = Reverse 1D Array(array=w576) -> (reversed array=w582:u8[])
                n1108 = Reverse 1D Array(array=w574) -> (reversed array=w581:u8[])
                n1109 = Reverse 1D Array(array=w571) -> (reversed array=w573:u8[])
                n1110 = Type Cast(type=w568, x=w607) -> (*(type *) &x=→"电机1实际速度":i32)
                n1111 = Type Cast(type=w568, x=w604) -> (*(type *) &x=→"电机1实际电流":i32)
                n1112 = Type Cast(type=w568, x=w601) -> (*(type *) &x=→"电机1实际位置":i32)
                n1113 = Type Cast(type=w568, x=w598) -> (*(type *) &x=→"电机2实际速度":i32)
                n1114 = Type Cast(type=w568, x=w595) -> (*(type *) &x=→"电机2实际电流":i32)
                n1115 = Type Cast(type=w568, x=w592) -> (*(type *) &x=→"电机2实际位置":i32)
                n1116 = Type Cast(type=w568, x=w589) -> (*(type *) &x=→"电机1状态":i32)
                n1117 = Type Cast(type=w568, x=w577) -> (*(type *) &x=→"电机2状态":i32)
                n1118 = Type Cast(type=w568, x=w582) -> (*(type *) &x=→"母线电压":i32)
                n1119 = Type Cast(type=w568, x=w581) -> (*(type *) &x=→"电机1温度":i32)
                n1120 = Type Cast(type=w568, x=w573) -> (*(type *) &x=→"电机2温度":i32)
              }
              frame Default {
                # "指令码0x00,无效"
              }
            }
            n1121 = Add(x=w74, y=1.0) -> (x+y=→"数值 3":dbl)
            "布尔" <- FALSE ("布尔")
            "数值 4" <- w72
          }
        }
      }
    }
    n1122 = property on="打开/关闭串口" class="Bool (严格)"() -> ("Value"=w16:bool)  [unwired: 2 in, 2 out]
  }
  n1123 = VISA Close(VISA resource name=w5) -> ()  [unwired: 1 in, 1 out]
